vi "ActorPlugin-001-CreateInstructions.vi"(0 "FTW Actor Instance Configuration":string="{\n  \"Identity\": \"ActorName\",\n  \"InboxAddress\": \"tcp://127.0.0.1:*\",\n  \"PublisherAddress\": \"tcp://127.0.0.1:*\",\n  \"DebugEnableInboxLogging\": false,\n  \"DebugEnableJobLogging\": false,\n  \"DebugShowPanel\": false\n}", 11 "Error in":errorcluster) -> (15 "Error":errorcluster)   [LabVIEW 2013, in "ERP-CreateInstructions.lvclass"]
uses:
  Actors/ERP-Create Instructions Plugin/ERP-CreateInstructions/ERP-CreateInstructions.lvclass
  Actors/ERP-Create Instructions Plugin/Instruction Controls/Cntrl-CreateManuInstruction.ctl
  Actors/ERP-Create Instructions Plugin/Instruction Controls/Cntrl-UpdateInstruction.ctl
  Actors/ERP-Create Instructions Plugin/Instruction Controls/Cntrl-CreateInspectInstruction.ctl
  Actors/ERP-Create Instructions Plugin/Instruction Controls/Cntrl-CreateGeneralInstruction.ctl
  Actors/ERP-Create Instructions Plugin/Instruction Controls/Cntrl-Manufacturing.ctl
  Actors/ERP-Create Instructions Plugin/Instruction Controls/Cntrl-Inspection.ctl
  Actors/ERP-Create Instructions Plugin/Instruction Controls/Cntrl-GenericCenter.ctl
  Actors/ERP-Create Instructions Plugin/Instruction Controls/Cntrl-ClearStep.ctl
  Actors/ERP-Create Instructions Plugin/Instruction Controls/Cntrl-LoadInstruction.ctl
  Actors/ERP-Create Instructions Plugin/Instruction Controls/Cntrl-ChooseGeneralStep.ctl
  Actors/ERP-Create Instructions Plugin/Instruction Controls/Cntrl-RefreshTree.ctl
  Actors/ERP-Create Instructions Plugin/Instruction Controls/Cntrl-ClearAllSteps.ctl
  Actors/ERP-Create Instructions Plugin/Instruction Controls/Cntrl-DeleteTreeItem.ctl
  Actors/ERP-Create Instructions Plugin/ERP-CreateInstructions/ERP-CreateInstructions.lvclass/ERP-CreateInstructions.ctl
  ftw-dataflow/Actor/src/Instance/FTW-ActorInstance.lvclass
  ftw-dataflow/Actor/src/Message/Request/FTW-Message-IncomingRequest.lvclass
  ERP-ConfigPageNewFeather/PCert-ConfigPageNF.lvclass
  <vilib>/addons/_LabVIEW Style Book/Utilities/Style Book Utilities.lvlib
panel:
  in  "Manufacturing Center":T1
  in  "Inspection Center":T2
  in  "Generic Instruction Center":T3
  in  "Stop Button":bool
  in  "Tab Control -Main":T4(tab)
  in  "Refresh Manufacturing Tree":T5
  in  "Clear Manu Step#":T6
  in  "Go Back A Step - Manu":bool
  in  "Go to next step-Manu":bool
  in  "Manufacturing Tab Instructions":T7(tab)
  in  "Manufacturing-Part Number":string
  in  "Manufacturing-Mat":T8={"Get Material Instruction"="", "Path for Picture Material"=path "", "Path for Picture Material 2"=path "", "Path for Picture Material 3"=path "", "Path for Picture Material 4"=path "", "Path for Picture Material 5"=path "", "Path for Picture Material 6"=path "", "Path for Picture Material 7"=path "", "Step Number"="1", "General Instruction"=""}
  in  "Manufacturing-VisualInsp":T9={"Visual Inspection Instruction"="", "Path for Picture VisualInsp"=path "", "Path for Picture VisualInsp 2"=path "", "Path for Picture VisualInsp 3"=path "", "Path for Picture VisualInsp 4"=path "", "Path for Picture VisualInsp 5"=path "", "Path for Picture VisualInsp 6"=path "", "Path for Picture VisualInsp 7"=path "", "Step Number"="2", "General Instruction"=""}
  in  "Manufacturing-Assemble":T10={"Assemble Material as Required"="", "Path for Picture Assemble"=path "", "Path for Picture Assemble 2"=path "", "Path for Picture Assemble 3"=path "", "Path for Picture Assemble 4"=path "", "Path for Picture Assemble 5"=path "", "Path for Picture Assemble 6"=path "", "Path for Picture Assemble 7"=path "", "Step Number"="3", "General Instruction"=""}
  in  "Manufacturing-Laser":T11={"Laser Cutting Instructions"="", "Path for Picture Laser Cutting"=path "", "Path for Picture Laser Cutting 2"=path "", "Path for Picture Laser Cutting 3"=path "", "Path for Picture Laser Cutting 4"=path "", "Path for Picture Laser Cutting 5"=path "", "Path for Picture Laser Cutting 6"=path "", "Path for Picture Laser Cutting 7"=path "", "Step Number"="4", "General Instruction"=""}
  in  "Manufacturing-Cleaning":T12={"Cleaning Instructions"="", "Path for Picture Cleaning"=path "", "Path for Picture Cleaning 2"=path "", "Path for Picture Cleaning 3"=path "", "Path for Picture Cleaning 4"=path "", "Path for Picture Cleaning 5"=path "", "Path for Picture Cleaning 6"=path "", "Path for Picture Cleaning 7"=path "", "Step Number"="5", "General Instruction"=""}
  in  "Manufacturing-Label":T13={"Label Instructions"="", "Path for Picture Label"=path "", "Path for Picture Label 2"=path "", "Path for Picture Label 3"=path "", "Path for Picture Label 4"=path "", "Path for Picture Label 5"=path "", "Path for Picture Label 6"=path "", "Path for Picture Label 7"=path "", "Step Number"="6", "General Instruction"=""}
  in  "Manufacturing Tree - Instruction Sets":string(tree)
  in  "Create Manufacturing Instruction":T14
  in  "Update Manufacturing Instruction":T15
  in  "Load Manufacturing Instruction":T16
  in  "Choose General Step\nManufacturing":T17
  in  "Clear All Manu\nSteps":T18
  in  "Delete Manufacturing Instruction":T19
  in  "Delete Inspection Instruction":T19
  in  "Clear All Inspection\nSteps":T18
  in  "Refresh Inspection Tree":T5
  in  "Inspection Tab Instructions":T20(tab)
  in  "Inspection Part Number":string caption="Part Number Inspection"
  in  "Inspect-Visually Inspect":T21={"Visual Inspection Instruction"="", "Path for Picture Material"=path "", "Path for Picture Material 2"=path "", "Path for Picture Material 3"=path "", "Path for Picture Material 4"=path "", "Path for Picture Material 5"=path "", "Path for Picture Material 6"=path "", "Path for Picture Material 7"=path "", "Step Number"="1", "General Instruction"=""}
  in  "Inspect-Certified Material":T22={"Certified Material Instruction"="", "Path for Picture VisualInsp"=path "", "Path for Picture VisualInsp 2"=path "", "Path for Picture VisualInsp 3"=path "", "Path for Picture VisualInsp 4"=path "", "Path for Picture VisualInsp 5"=path "", "Path for Picture VisualInsp 6"=path "", "Path for Picture VisualInsp 7"=path "", "Step Number"="2", "General Instruction"=""}
  in  "Inspect-XY Dimensions":T23={"XY Dimensions Instructions"="", "Path for Picture Assemble"=path "", "Path for Picture Assemble 2"=path "", "Path for Picture Assemble 3"=path "", "Path for Picture Assemble 4"=path "", "Path for Picture Assemble 5"=path "", "Path for Picture Assemble 6"=path "", "Path for Picture Assemble 7"=path "", "Step Number"="3", "General Instruction"=""}
  in  "Inspect-Measure Create Cert":T24={"Measure and Create Certification Instructions"="", "Path for Picture Laser Cutting"=path "", "Path for Picture Laser Cutting 2"=path "", "Path for Picture Laser Cutting 3"=path "", "Path for Picture Laser Cutting 4"=path "", "Path for Picture Laser Cutting 5"=path "", "Path for Picture Laser Cutting 6"=path "", "Path for Picture Laser Cutting 7"=path "", "Step Number"="4", "General Instruction"=""}
  in  "Inspect-Qty P/F":T25={"Quantity Passed or Failed Instructions"="", "Path for Picture Cleaning"=path "", "Path for Picture Cleaning 2"=path "", "Path for Picture Cleaning 3"=path "", "Path for Picture Cleaning 4"=path "", "Path for Picture Cleaning 5"=path "", "Path for Picture Cleaning 6"=path "", "Path for Picture Cleaning 7"=path "", "Step Number"="5", "General Instruction"=""}
  in  "Inspect-Inspect Labels":T26={"Inspect Label Instructions"="", "Path for Picture Label"=path "", "Path for Picture Label 2"=path "", "Path for Picture Label 3"=path "", "Path for Picture Label 4"=path "", "Path for Picture Label 5"=path "", "Path for Picture Label 6"=path "", "Path for Picture Label 7"=path "", "Step Number"="6", "General Instruction"=""}
  in  "Inspection Tree - Instruction Sets":string(tree)
  in  "Go to next step-Insp":bool
  in  "Go Back A Step - Insp":bool
  in  "Create Inspection Instruction":T27
  in  "Clear Inspect Step#":T6
  in  "Load Inspection Instruction":T16
  in  "Update Inspection Instruction":T15
  in  "Choose General Step\nInspection":T17
  in  "Step Number*":dbl
  in  "General Process Name*":string
  in  "General Tree - Instruction Sets":string(tree)
  in  "Create General Instruction":T28
  in  "General Step Instruction":T29
  in  "Clear General Step#":T6
  in  "Refresh General Tree":T5
  in  "Update General Instruction":T15
  in  "Delete General Instruction":T19
  # "Instruction Controls"
  # "Inputs"
  # "Outputs"
  # "Please Enter the Part Number"
  # "Enter Instruction for Get Material"
  # "Enter Instruction Visual Inspection"
  # "Enter Instruction for Assemble Material as Required"
  # "Enter Instruction for Laser Cutting"
  # "Enter Instruction for Cleaning"
  # "Enter Instruction for Label"
  # "Please Enter the Part Number"
  # "Enter Instruction for Visually Inspect"
  # "Enter Instruction Verify Certified Material Was Used"
  # "Enter Instruction for Verify XY Dimensions"
  # "Enter Instruction Measure: Create Certification if Required"
  # "Enter Instruction For Verify Quantity Passed or Failed"
  # "Enter Instruction for Label Inspection"
  # "General Instuctions"
  # "*=Required"
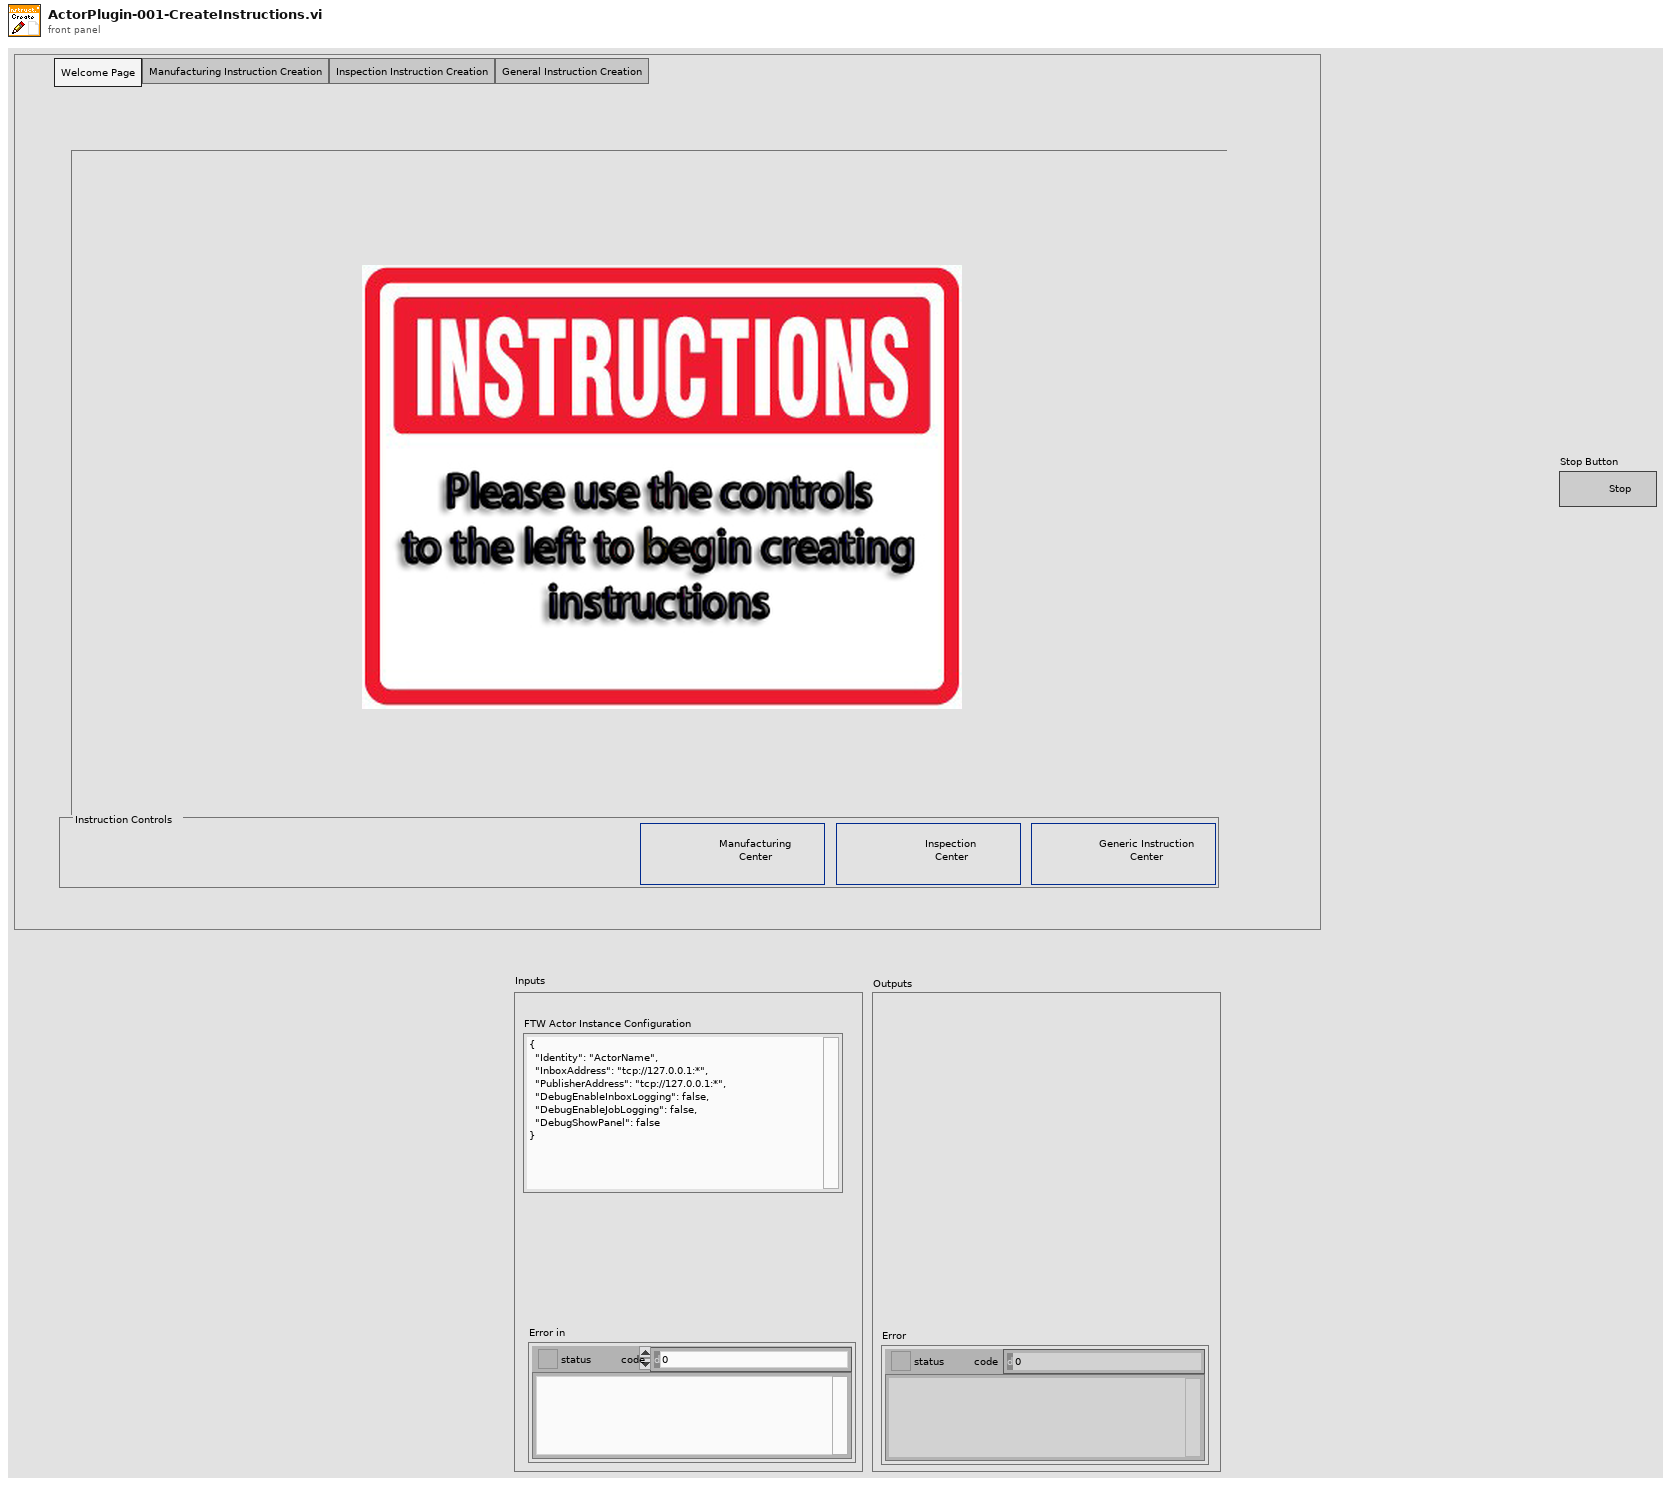
[diagram p1: front panel]
types:
  T1 = typedef "Cntrl-Manufacturing.ctl" = bool
  T2 = typedef "Cntrl-Inspection.ctl" = bool
  T3 = typedef "Cntrl-GenericCenter.ctl" = bool
  T4 = enum32{"Welcome Page", "Manufacturing Instruction Creation", "Inspection Instruction Creation", "General Instruction Creation"}
  T5 = typedef "Cntrl-RefreshTree.ctl" = bool
  T6 = typedef "Cntrl-ClearStep.ctl" = bool
  T7 = enum32{"Enter Part Number", "Get Material Instructions", "Visual Inspection Instruction", "Assemble Material as Required", "Laser Cutting Instructions", "Cleaning Instructions", "Label Instructions"}
  T8 = cluster{"Get Material Instruction":string, "Path for Picture Material":path, "Path for Picture Material 2":path, "Path for Picture Material 3":path, "Path for Picture Material 4":path, "Path for Picture Material 5":path, "Path for Picture Material 6":path, "Path for Picture Material 7":path, "Step Number":string, "General Instruction":string}
  T9 = cluster{"Visual Inspection Instruction":string, "Path for Picture VisualInsp":path, "Path for Picture VisualInsp 2":path, "Path for Picture VisualInsp 3":path, "Path for Picture VisualInsp 4":path, "Path for Picture VisualInsp 5":path, "Path for Picture VisualInsp 6":path, "Path for Picture VisualInsp 7":path, "Step Number":string, "General Instruction":string}
  T10 = cluster{"Assemble Material as Required":string, "Path for Picture Assemble":path, "Path for Picture Assemble 2":path, "Path for Picture Assemble 3":path, "Path for Picture Assemble 4":path, "Path for Picture Assemble 5":path, "Path for Picture Assemble 6":path, "Path for Picture Assemble 7":path, "Step Number":string, "General Instruction":string}
  T11 = cluster{"Laser Cutting Instructions":string, "Path for Picture Laser Cutting":path, "Path for Picture Laser Cutting 2":path, "Path for Picture Laser Cutting 3":path, "Path for Picture Laser Cutting 4":path, "Path for Picture Laser Cutting 5":path, "Path for Picture Laser Cutting 6":path, "Path for Picture Laser Cutting 7":path, "Step Number":string, "General Instruction":string}
  T12 = cluster{"Cleaning Instructions":string, "Path for Picture Cleaning":path, "Path for Picture Cleaning 2":path, "Path for Picture Cleaning 3":path, "Path for Picture Cleaning 4":path, "Path for Picture Cleaning 5":path, "Path for Picture Cleaning 6":path, "Path for Picture Cleaning 7":path, "Step Number":string, "General Instruction":string}
  T13 = cluster{"Label Instructions":string, "Path for Picture Label":path, "Path for Picture Label 2":path, "Path for Picture Label 3":path, "Path for Picture Label 4":path, "Path for Picture Label 5":path, "Path for Picture Label 6":path, "Path for Picture Label 7":path, "Step Number":string, "General Instruction":string}
  T14 = typedef "Cntrl-CreateManuInstruction.ctl" = bool
  T15 = typedef "Cntrl-UpdateInstruction.ctl" = bool
  T16 = typedef "Cntrl-LoadInstruction.ctl" = bool
  T17 = typedef "Cntrl-ChooseGeneralStep.ctl" = bool
  T18 = typedef "Cntrl-ClearAllSteps.ctl" = bool
  T19 = typedef "Cntrl-DeleteTreeItem.ctl" = bool
  T20 = enum32{"Enter Part Number", "Visually Inspect", "Certified Material", "XY Dimensions", "Measure Create Cert", "Quantity Passed or Failed", "Inspect Labels"}
  T21 = cluster{"Visual Inspection Instruction":string, "Path for Picture Material":path, "Path for Picture Material 2":path, "Path for Picture Material 3":path, "Path for Picture Material 4":path, "Path for Picture Material 5":path, "Path for Picture Material 6":path, "Path for Picture Material 7":path, "Step Number":string, "General Instruction":string}
  T22 = cluster{"Certified Material Instruction":string, "Path for Picture VisualInsp":path, "Path for Picture VisualInsp 2":path, "Path for Picture VisualInsp 3":path, "Path for Picture VisualInsp 4":path, "Path for Picture VisualInsp 5":path, "Path for Picture VisualInsp 6":path, "Path for Picture VisualInsp 7":path, "Step Number":string, "General Instruction":string}
  T23 = cluster{"XY Dimensions Instructions":string, "Path for Picture Assemble":path, "Path for Picture Assemble 2":path, "Path for Picture Assemble 3":path, "Path for Picture Assemble 4":path, "Path for Picture Assemble 5":path, "Path for Picture Assemble 6":path, "Path for Picture Assemble 7":path, "Step Number":string, "General Instruction":string}
  T24 = cluster{"Measure and Create Certification Instructions":string, "Path for Picture Laser Cutting":path, "Path for Picture Laser Cutting 2":path, "Path for Picture Laser Cutting 3":path, "Path for Picture Laser Cutting 4":path, "Path for Picture Laser Cutting 5":path, "Path for Picture Laser Cutting 6":path, "Path for Picture Laser Cutting 7":path, "Step Number":string, "General Instruction":string}
  T25 = cluster{"Quantity Passed or Failed Instructions":string, "Path for Picture Cleaning":path, "Path for Picture Cleaning 2":path, "Path for Picture Cleaning 3":path, "Path for Picture Cleaning 4":path, "Path for Picture Cleaning 5":path, "Path for Picture Cleaning 6":path, "Path for Picture Cleaning 7":path, "Step Number":string, "General Instruction":string}
  T26 = cluster{"Inspect Label Instructions":string, "Path for Picture Label":path, "Path for Picture Label 2":path, "Path for Picture Label 3":path, "Path for Picture Label 4":path, "Path for Picture Label 5":path, "Path for Picture Label 6":path, "Path for Picture Label 7":path, "Step Number":string, "General Instruction":string}
  T27 = typedef "Cntrl-CreateInspectInstruction.ctl" = bool
  T28 = typedef "Cntrl-CreateGeneralInstruction.ctl" = bool
  T29 = cluster{"General Instruction Step":string, "Path for Picture General":path, "Path for Picture General 2":path, "Path for Picture General 3":path, "Path for Picture General 4":path, "Path for Picture General 5":path, "Path for Picture General 6":path, "Path for Picture General 7":path}
  T30 = cluster{"Manufacturing-Part Number":string, dbl, "Manufacturing-Label":cluster{"Label Instructions":string, "Path for Picture Label":path, "Path for Picture Label 2":path, "Path for Picture Label 3":path, "Path for Picture Label 4":path, "Path for Picture Label 5":path, "Path for Picture Label 6":path, "Path for Picture Label 7":path}}
  T31 = enum32{"Welcome Page", "Manufacturing Instruction Creation", "Inspection Instruction Creation"}
  T32 = cluster{"Manufacturing-Part Number":string, "Array of Cluster Data":cluster{"Label Instructions":string, "Path for Picture Label":path, "Path for Picture Label 2":path, "Path for Picture Label 3":path, "Path for Picture Label 4":path, "Path for Picture Label 5":path, "Path for Picture Label 6":path, "Path for Picture Label 7":path, "Label Instructions 2":string, "Label Instructions 3":string}[], "Type of Insert":i32}
  T33 = cluster{"Manufacturing-Part Number":string, "Step Number":dbl, "Gernal Cluster Data":cluster{"Label Instructions":string, "Path for Picture Label":path, "Path for Picture Label 2":path, "Path for Picture Label 3":path, "Path for Picture Label 4":path, "Path for Picture Label 5":path, "Path for Picture Label 6":path, "Path for Picture Label 7":path}, "Type of Insert":i32}
  T34 = cluster{"Label Instructions":string, "Path for Picture Label":path, "Path for Picture Label 2":path, "Path for Picture Label 3":path, "Path for Picture Label 4":path, "Path for Picture Label 5":path, "Path for Picture Label 6":path, "Path for Picture Label 7":path, "Step Number":string, "General Instruction":string}[]
  T35 = cluster{"Value":string, cluster{"Label Instructions":string, "Path for Picture Label":path, "Path for Picture Label 2":path, "Path for Picture Label 3":path, "Path for Picture Label 4":path, "Path for Picture Label 5":path, "Path for Picture Label 6":path, "Path for Picture Label 7":path, "Step Number":string, "General Instruction":string}[]}
  T36 = cluster{"Inspect Label Instructions":string, "Path for Picture Label":path, "Path for Picture Label 2":path, "Path for Picture Label 3":path, "Path for Picture Label 4":path, "Path for Picture Label 5":path, "Path for Picture Label 6":path, "Path for Picture Label 7":path, "Step Number":string, "General Instruction":string}[]
  T37 = cluster{"Value":string, cluster{"Inspect Label Instructions":string, "Path for Picture Label":path, "Path for Picture Label 2":path, "Path for Picture Label 3":path, "Path for Picture Label 4":path, "Path for Picture Label 5":path, "Path for Picture Label 6":path, "Path for Picture Label 7":path, "Step Number":string, "General Instruction":string}[]}
  T38 = cluster{"Incoming Requests":refnum<event-registration>, "Additional Registration Types":refnum<event-registration>}
  T39 = cluster{"Label Instructions":string, "Path for Picture Label":path, "Path for Picture Label 2":path, "Path for Picture Label 3":path, "Path for Picture Label 4":path, "Path for Picture Label 5":path, "Path for Picture Label 6":path, "Path for Picture Label 7":path, "Step Number":string, "Generall Instruction":string}[]
  T40 = cluster{"Label Instructions":string, "Path for Picture Label":path, "Path for Picture Label 2":path, "Path for Picture Label 3":path, "Path for Picture Label 4":path, "Path for Picture Label 5":path, "Path for Picture Label 6":path, "Path for Picture Label 7":path}
  T41 = cluster{"Instructions":string, "Picture Path 1":path, "Picture Path 2":path, "Picture Path 3":path, "Picture Path 4":path, "Picture Path 5":path, "Picture Path 6":path, "Picture Path 7":path, "Step":string, "General Instruction":string}[]
  T42 = cluster{"Instructions":string, "Picture Path 1":path, "Picture Path 2":path, "Picture Path 3":path, "Picture Path 4":path, "Picture Path 5":path, "Picture Path 6":path, "Picture Path 7":path, "Step":string, "General Instrucion":string}
  T43 = cluster{"Instructions":string, "Picture Path 1":path, "Picture Path 2":path, "Picture Path 3":path, "Picture Path 4":path, "Picture Path 5":path, "Picture Path 6":path, "Picture Path 7":path, "Step Instruction":string, "General Instruction":string}
  T44 = cluster{"Instructions":string, "Picture Path 1":path, "Picture Path 2":path, "Picture Path 3":path, "Picture Path 4":path, "Picture Path 5":path, "Picture Path 6":path, "Picture Path 7":path}
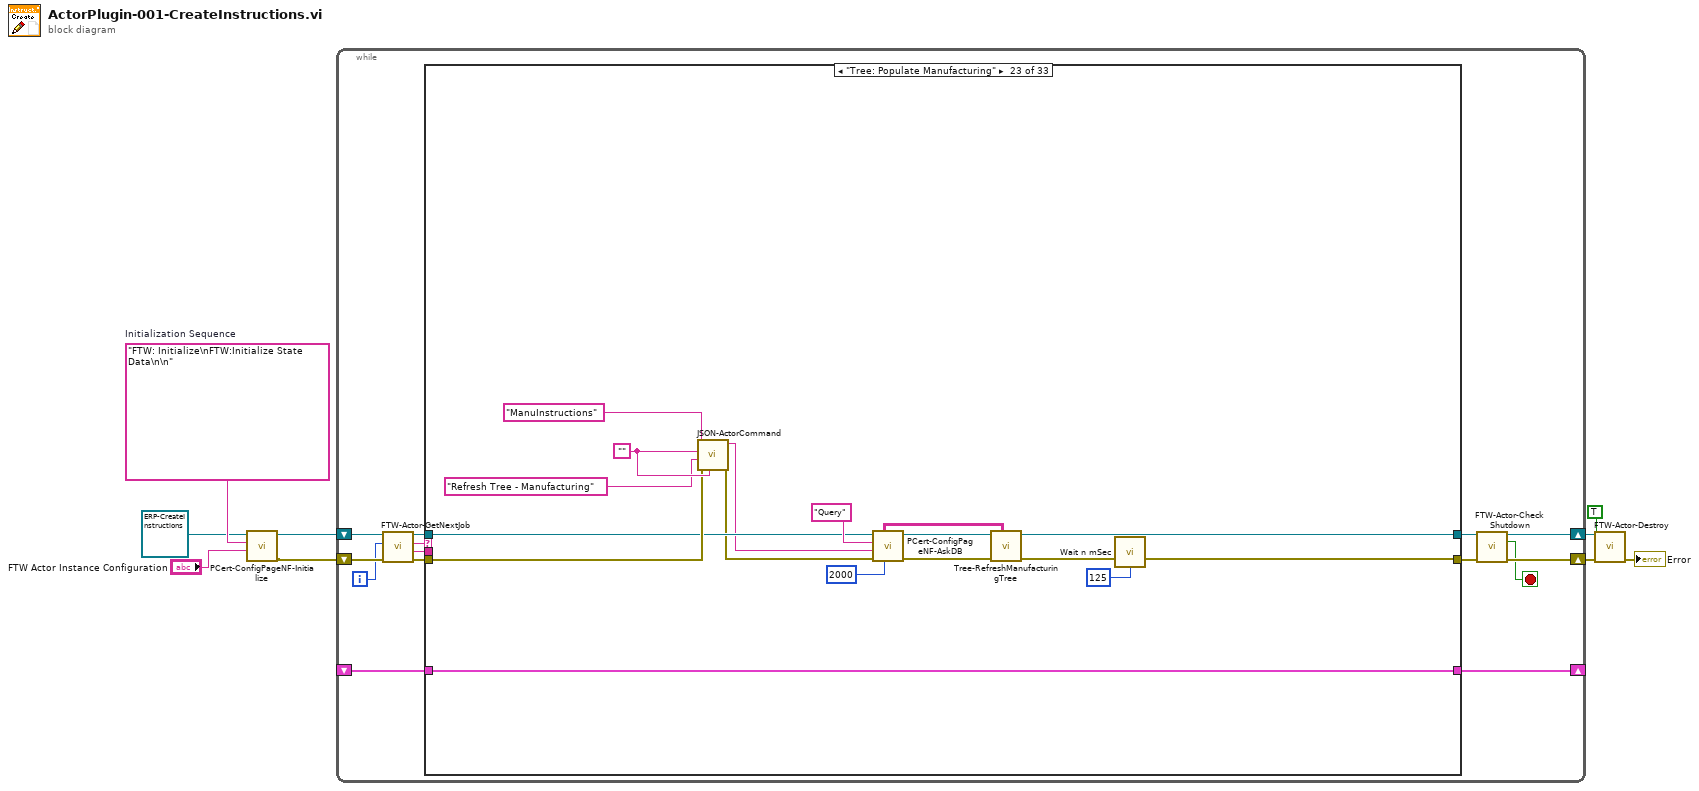
[diagram p0: block diagram]
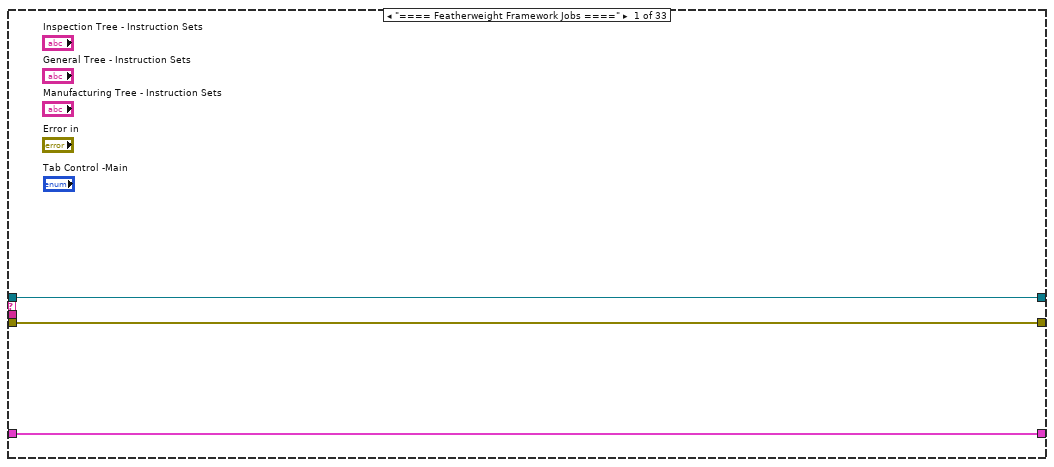
[diagram p2: hidden frame]
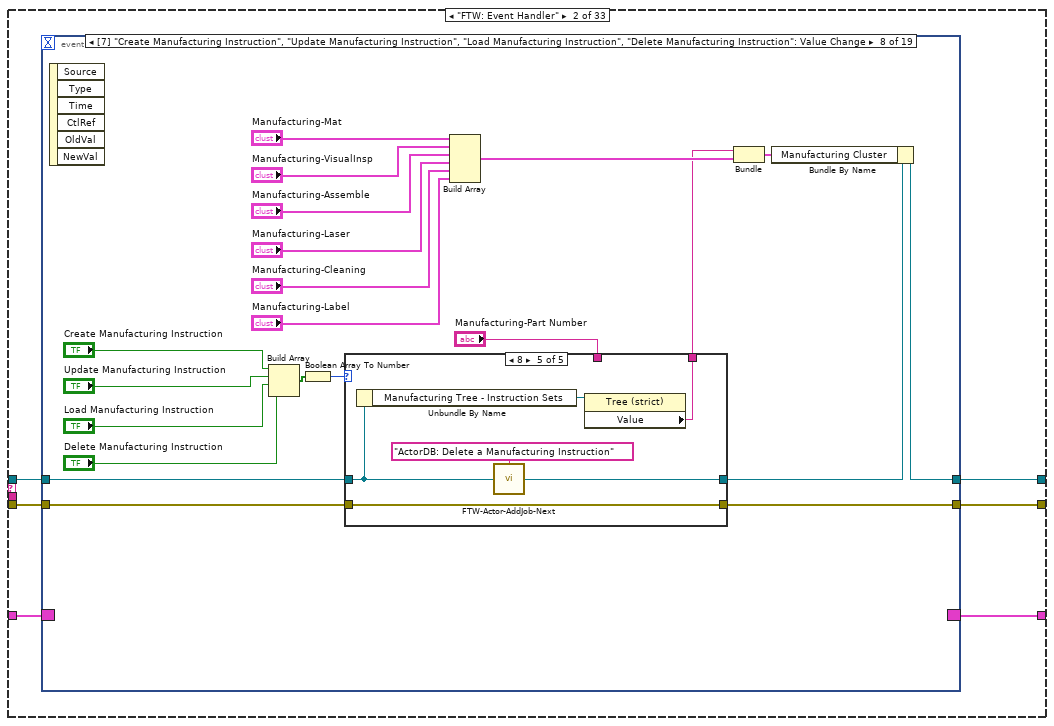
[diagram p3: hidden frame]
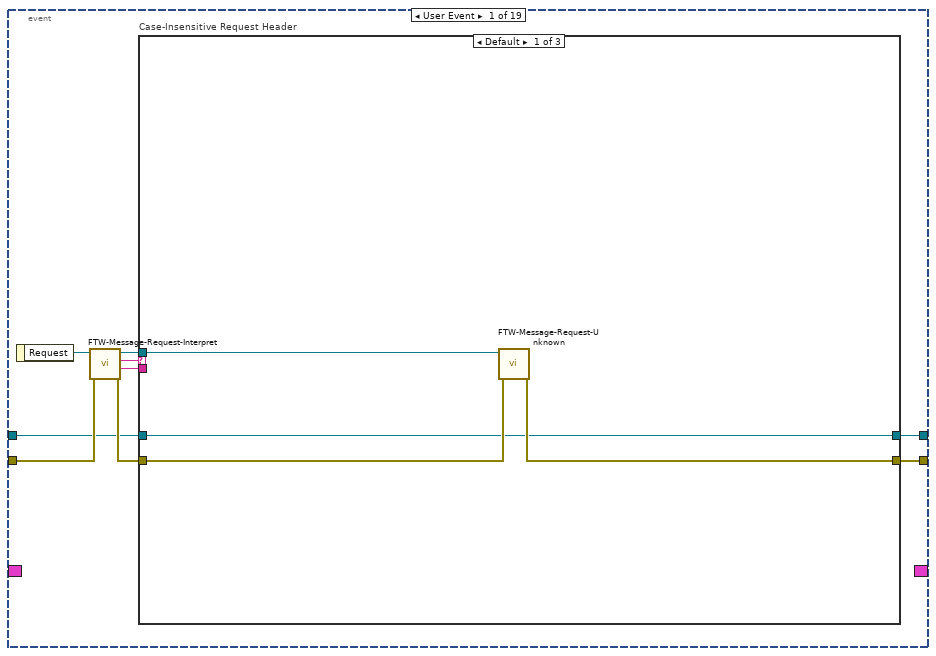
[diagram p4: hidden frame]
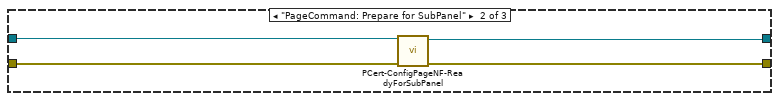
[diagram p5: hidden frame]
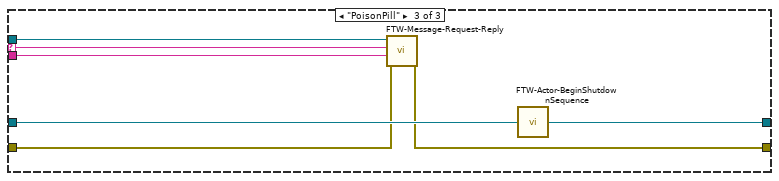
[diagram p6: hidden frame]
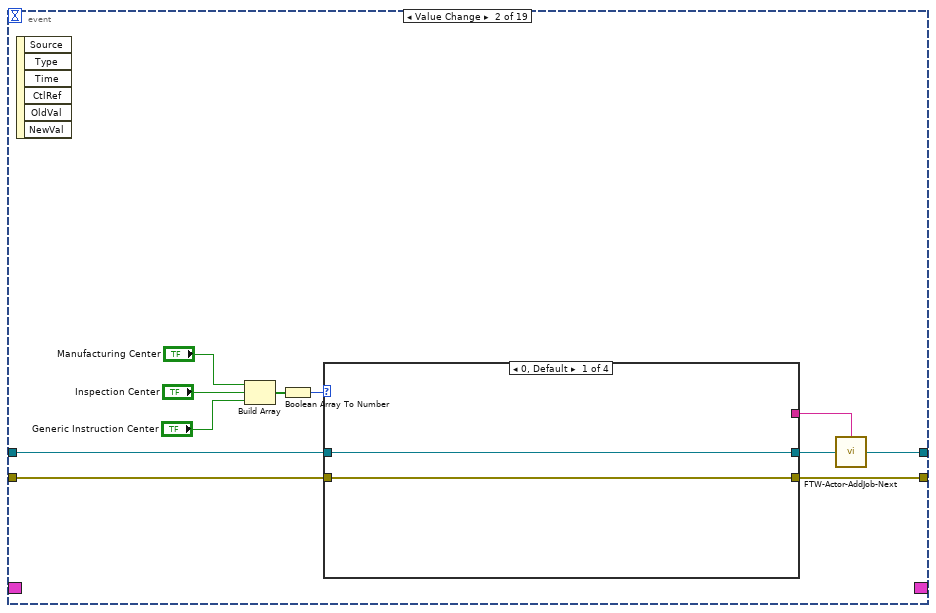
[diagram p7: hidden frame]
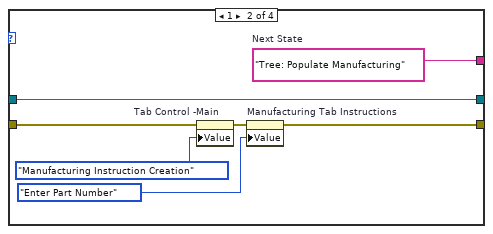
[diagram p8: hidden frame]
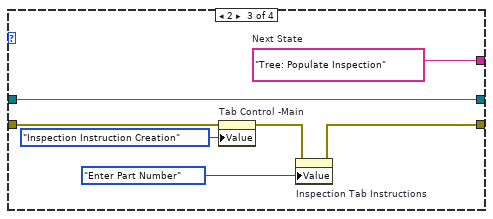
[diagram p9: hidden frame]
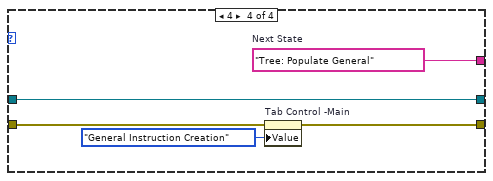
[diagram p10: hidden frame]
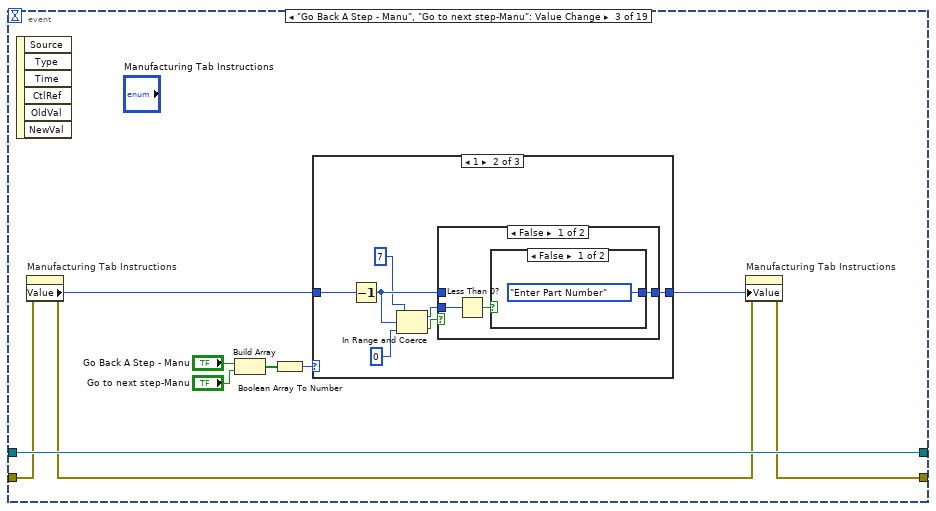
[diagram p11: hidden frame]
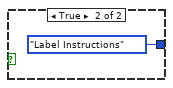
[diagram p13: hidden frame]
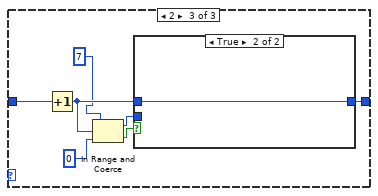
[diagram p15: hidden frame]
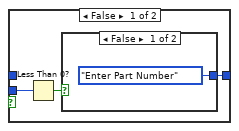
[diagram p16: hidden frame]
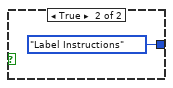
[diagram p17: hidden frame]
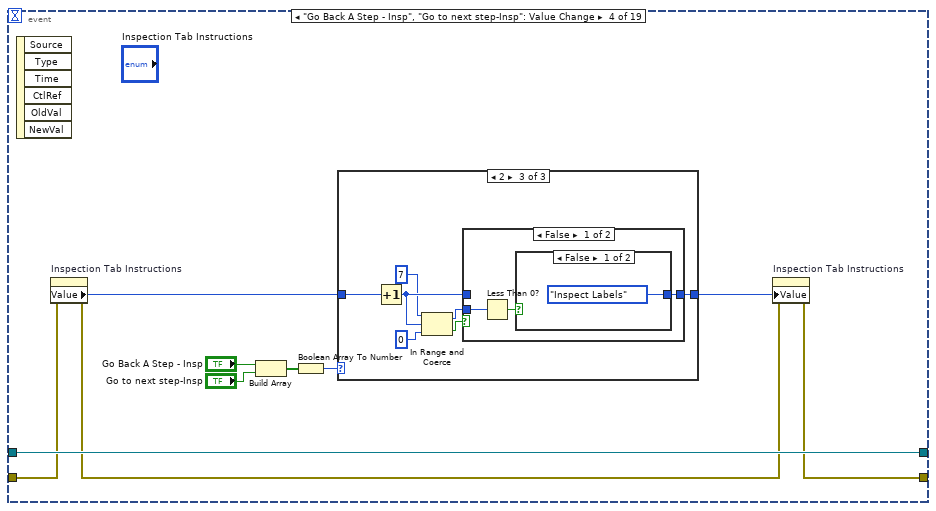
[diagram p18: hidden frame]
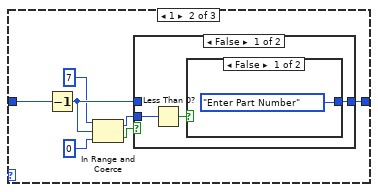
[diagram p20: hidden frame]
diagram:
  w6 = "FTW: Initialize\nFTW:Initialize State Data\n\n"  # Initialization Sequence
  n1 = call-dynamic "PCert-ConfigPageNF-Initialize.vi"("FTW Actor Instance Configuration"="FTW Actor Instance Configuration", "Initialization Job Sequence"=w6, "ERP-ConfigPageNF.lvclass"=refnum<class "ERP-CreateInstructions.lvclass"> refnum ("ERP-CreateInstructions.lvclass")) -> ("error out"=w4:errorcluster, "ERP-ConfigPageNF out"=w5:refnum<class "ERP-CreateInstructions.lvclass">)  [unwired: 7 in]
  n2 = while {
    shift-right: [w13] -> w8
    shift-left: w4 -> [w20]
    shift-right: [w10] -> _
    shift-left: _ -> [w23]
    shift-right: [w15] -> w9
    shift-left: w5 -> [w22]
    i -> [w11]
    stop <- w12 stop-if-true
    n3 = call "FTW-Actor-GetNextJob.vi"("error in"=w20, "Jobs Performed"=w11, "FTW Actor Instance"=w22) -> ("error out"=w19:errorcluster, "Job Data"=w17:string, "Job Name"=w18:string, "FTW Actor Instance out"=w21:refnum<class "ERP-CreateInstructions.lvclass">)  [unwired: 5 in]
    n4 = case shown="\"Tree: Populate Manufacturing\"" w18 {
      selector: w18 -> [_ _ _ _ _ w435 _ _ _ _ _ _ _ _ _ _ _ _ _ _ _ _ _ _ _ _ _ _ _ _ _ _ _]
      tunnel: [w25 w32 w418 w428 w430 w438 w446 w452 w457 w461 w465 w491 w510 w534 w558 w580 w606 w639 w682 w698 w723 w755 w757 w774 w791 w808 w811 w814 w873 w919 w931 w945 w997] -> w14
      tunnel: w19 -> [w25 w31 w410 w428 w432 w439 w443 w452 w457 w461 w462 w485 w519 w532 w556 w590 w615 w648 w684 w712 w733 w755 w769 w786 w803 w808 w811 w821 w871 w926 w931 w936 w1001]
      tunnel: w23 -> [w26 w27 _ w429 w434 w440 w448 w453 w458 w460 w484 w507 w531 w555 w579 w604 w616 w650 w697 w722 w751 w756 w773 w790 w807 w810 w813 w822 w874 w929 w932 w948 w1009]
      tunnel: [w26 w30 w412 w429 w434 w440 w448 w453 w458 w460 w484 w507 w531 w555 w579 w604 w616 w650 w697 w722 w751 w756 w773 w790 w807 w810 w813 w822 w874 w929 w932 w948 w1009] -> w10
      tunnel: w17 -> [_ _ _ _ _ _ _ _ _ _ _ _ _ _ _ _ _ _ _ _ _ _ _ _ _ _ _ _ _ _ _ _ _]
      tunnel: [w24 w29 w419 w425 w431 w436 w441 w450 w455 w459 w466 w492 w511 w535 w559 w581 w613 w646 w683 w699 w727 w754 w760 w777 w794 w809 w812 w818 w868 w928 w930 w944 w998] -> w16
      tunnel: w21 -> [w24 w28 w417 w427 w433 w437 w444 w451 w456 w459 w463 w486 w515 w533 w557 w587 w614 w647 w681 w711 w746 w754 w766 w783 w800 w809 w812 w820 w872 w927 w930 w937 w1002]
      frame "==== Featherweight Framework Jobs ====" {
      }
      frame "FTW: Event Handler" {
        n5 = event shown="[7] \"Create Manufacturing Instruction\", \"Update Manufacturing Instruction\", \"Load Manufacturing Instruction\", \"Delete Manufacturing Instruction\": Value Change" {
          selector: w27 -> [_ _ _ _ _ _ _ _ _ _ _ _ _ _ _ _ _ _ _]
          dyn-events: [_ _ _ _ _ _ _ _ _ _ _ _ _ _ _ _ _ _ _] -> w30
          timeout: _ -> [_ _ _ _ _ _ _ _ _ _ _ _ _ _ _ _ _ _ _]
          tunnel: [w38 w66 w97 w132 w163 w182 w201 w219 w254 w258 w273 w304 w311 w312 w336 w366 w400 w403 w406] -> w32
          tunnel: w31 -> [w39 w67 w96 w134 w166 w185 w202 w226 w254 w258 w274 w304 w311 w313 w337 w371 w400 w403 w406]
          tunnel: [w37 w58 w98 w135 w167 w186 w205 w210 w251 w255 w271 w305 w308 w314 w335 w373 w397 w401 w404] -> w29
          tunnel: w28 -> [w36 w62 w98 w135 w167 w186 w205 w225 w252 w256 w275 w306 w309 w315 w335 w372 w398 w402 w405]
          event User Event {
            n6 = event-data() -> ("Request"=w40:refnum<class "FTW-Message-IncomingRequest.lvclass">)  [unwired: 1 in]
            n7 = call "FTW-Message-Request-Interpret.vi"("error in"=w39, "FTW Incoming Request"=w40) -> ("error out"=w41:errorcluster, "Request Body"=w34:string, "Request Header"=w35:string, "FTW Incoming Request out"=w33:refnum<class "FTW-Message-IncomingRequest.lvclass">)  [unwired: 6 in]
            n8 = case "Case-Insensitive Request Header" shown="Default" w35 {
              selector: w35 -> [_ _ w52]
              tunnel: [w44 w46 w50] -> w38
              tunnel: w41 -> [w45 w47 w51]
              tunnel: [w42 w48 w56] -> w37
              tunnel: w36 -> [w42 w49 w55]
              tunnel: w34 -> [_ _ w53]
              tunnel: w33 -> [w43 _ w54]
              frame Default {
                n9 = call "FTW-Message-Request-Unknown.vi"("error in"=w45, "FTW Incoming Request"=w43) -> ("error out"=w44:errorcluster)  [unwired: 9 in]
              }
              frame "PageCommand: Prepare for SubPanel" {
                n10 = call "PCert-ConfigPageNF-ReadyForSubPanel.vi"("error in (no error)"=w47, "ERP-ConfigPageNF in"=w49) -> ("error out"=w46:errorcluster, "ERP-ConfigPageNF out"=w48:refnum<class "ERP-CreateInstructions.lvclass">)  [unwired: 8 in]
              }
              frame "PoisonPill" {
                n11 = call "FTW-Message-Request-Reply.vi"("error in"=w51, "Response Body"=w53, "Response Header"=w52, "FTW Incoming Request"=w54) -> ("error out"=w50:errorcluster)  [unwired: 6 in, 1 out]
                n12 = call "FTW-Actor-BeginShutdownSequence.vi"("FTW Actor Instance"=w55) -> ("FTW Actor Instance out"=w56:refnum<class "ERP-CreateInstructions.lvclass">)  [unwired: 3 in]
              }
            }
          }
          event Value Change {
            n13 = event-data() -> ()  [unwired: 1 in, 6 out]
            n14 = Build Array("Manufacturing Center", "Inspection Center", "Generic Instruction Center") -> (w61:T3[])
            n15 = Boolean Array To Number(Boolean array=w61) -> (number=w60:u32)
            n16 = case shown="0, Default" w60 {
              tunnel: w67 -> [w68 w76 w83 w88]
              tunnel: [w68 w71 w77 w87] -> w66
              tunnel: w62 -> [w69 w74 w81 w85]
              tunnel: [w69 w74 w81 w85] -> w59
              tunnel: [_ w70 w80 w84] -> w57
              frame 0, Default {
              }
              frame 1 {
                w70 = "Tree: Populate Manufacturing"  # Next State
                n17 = property on="Tab Control -Main" class="TabCtl (strict)"(error in=w76, "Value"=T4."Manufacturing Instruction Creation" ("Tab Control -Main")) -> (error out=w72:errorcluster)  [unwired: 1 in, 1 out]
                n18 = property on="Manufacturing Tab Instructions" class="TabCtl (strict)"(error in=w72, "Value"=T7."Enter Part Number" ("Manufacturing Tab Instructions")) -> (error out=w71:errorcluster)  [unwired: 1 in, 1 out]
              }
              frame 2 {
                w80 = "Tree: Populate Inspection"  # Next State
                n19 = property on="Tab Control -Main" class="TabCtl (strict)"(error in=w83, "Value"=T4."Inspection Instruction Creation" ("Tab Control -Main")) -> (error out=w78:errorcluster)  [unwired: 1 in, 1 out]
                n20 = property on="Inspection Tab Instructions" class="TabCtl (strict)"(error in=w78, "Value"=T20."Enter Part Number" ("Inspection Tab Instructions")) -> (error out=w77:errorcluster)  [unwired: 1 in, 1 out]
              }
              frame 4 {
                w84 = "Tree: Populate General"  # Next State
                n21 = property on="Tab Control -Main" class="TabCtl (strict)"(error in=w88, "Value"=T4."General Instruction Creation" ("Tab Control -Main")) -> (error out=w87:errorcluster)  [unwired: 1 in, 1 out]
              }
            }
            n22 = call "FTW-Actor-AddJob-Next.vi"("Add Next in Job Queue"=w57, "FTW Actor Instance"=w59) -> ("FTW Actor Instance out"=w58:refnum<class "ERP-CreateInstructions.lvclass">)  [unwired: 2 in]
          }
          event "Go Back A Step - Manu", "Go to next step-Manu": Value Change {
            n23 = event-data() -> ()  [unwired: 1 in, 6 out]
            n24 = property on="Manufacturing Tab Instructions" class="TabCtl (strict)"(error in=w96) -> (error out=w95:errorcluster, "Value"=w90:T7)  [unwired: 1 in, 1 out]
            n25 = Build Array("Go Back A Step - Manu", "Go to next step-Manu") -> (w92:bool[])
            n26 = Boolean Array To Number(Boolean array=w92) -> (number=w91:u32)
            n27 = case shown="1" w91 {
              tunnel: w90 -> [w99 w106 w116]
              tunnel: [w99 w105 w115] -> w89
              frame 0, Default {
              }
              frame 1 {
                n28 = Decrement(x=w106) -> (x-1=w104:T7)
                n29 = In Range and Coerce(upper limit=7, x=w104, lower limit=0) -> (coerced(x)=w102:u32, In Range?=w103:bool)
                n30 = case shown="False" w103 {
                  tunnel: w104 -> [_ w112]
                  tunnel: [w107 w112] -> w105
                  tunnel: w102 -> [w109 _]
                  frame False {
                    n31 = Less Than 0?(x=w109) -> (x < 0?=w108:bool)
                    n32 = case shown="False" w108 {
                      tunnel: [T7."Enter Part Number" ("lower limit") T7."Label Instructions" ("lower limit")] -> w107
                      frame False {
                      }
                      frame True {
                      }
                    }
                  }
                  frame True {
                  }
                }
              }
              frame 2 {
                n33 = Increment(x=w116) -> (x+1=w119:T7)
                n34 = In Range and Coerce(upper limit=7, x=w119, lower limit=0) -> (coerced(x)=w117:u32, In Range?=w118:bool)
                n35 = case shown="True" w118 {
                  tunnel: w119 -> [_ w125]
                  tunnel: [w120 w125] -> w115
                  tunnel: w117 -> [w122 _]
                  frame False {
                    n36 = Less Than 0?(x=w122) -> (x < 0?=w121:bool)
                    n37 = case shown="False" w121 {
                      tunnel: [T7."Enter Part Number" ("lower limit") T7."Label Instructions" ("lower limit")] -> w120
                      frame False {
                      }
                      frame True {
                      }
                    }
                  }
                  frame True {
                  }
                }
              }
            }
            n38 = property on="Manufacturing Tab Instructions" class="TabCtl (strict)"(error in=w95, "Value"=w89) -> (error out=w97:errorcluster)  [unwired: 1 in, 1 out]
          }
          event "Go Back A Step - Insp", "Go to next step-Insp": Value Change {
            n39 = event-data() -> ()  [unwired: 1 in, 6 out]
            n40 = property on="Inspection Tab Instructions" class="TabCtl (strict)"(error in=w134) -> (error out=w133:errorcluster, "Value"=w131:T20)  [unwired: 1 in, 1 out]
            n41 = Build Array("Go Back A Step - Insp", "Go to next step-Insp") -> (w130:bool[])
            n42 = Boolean Array To Number(Boolean array=w130) -> (number=w128:u32)
            n43 = case shown="2" w128 {
              tunnel: w131 -> [w136 w143 w153]
              tunnel: [w136 w142 w152] -> w126
              frame 0, Default {
              }
              frame 1 {
                n44 = Decrement(x=w143) -> (x-1=w141:T20)
                n45 = In Range and Coerce(upper limit=7, x=w141, lower limit=0) -> (coerced(x)=w139:u32, In Range?=w140:bool)
                n46 = case shown="False" w140 {
                  tunnel: w141 -> [_ w149]
                  tunnel: [w144 w149] -> w142
                  tunnel: w139 -> [w146 _]
                  frame False {
                    n47 = Less Than 0?(x=w146) -> (x < 0?=w145:bool)
                    n48 = case shown="False" w145 {
                      tunnel: [T20."Enter Part Number" ("Inspection Tab Instructions") T20."Inspect Labels" ("Inspection Tab Instructions")] -> w144
                      frame False {
                      }
                      frame True {
                      }
                    }
                  }
                  frame True {
                  }
                }
              }
              frame 2 {
                n49 = Increment(x=w153) -> (x+1=w156:T20)
                n50 = In Range and Coerce(upper limit=7, x=w156, lower limit=0) -> (coerced(x)=w154:u32, In Range?=w155:bool)
                n51 = case shown="False" w155 {
                  tunnel: w156 -> [_ w162]
                  tunnel: [w157 w162] -> w152
                  tunnel: w154 -> [w159 _]
                  frame False {
                    n52 = Less Than 0?(x=w159) -> (x < 0?=w158:bool)
                    n53 = case shown="False" w158 {
                      tunnel: [T20."Inspect Labels" ("Inspection Tab Instructions") T20."Enter Part Number" ("Inspection Tab Instructions")] -> w157
                      frame False {
                      }
                      frame True {
                      }
                    }
                  }
                  frame True {
                  }
                }
              }
            }
            n54 = property on="Inspection Tab Instructions" class="TabCtl (strict)"(error in=w133, "Value"=w126) -> (error out=w132:errorcluster)  [unwired: 1 in, 1 out]
          }
          event Value Change {
            n55 = event-data() -> ()  [unwired: 1 in, 6 out]
            n56 = property on="Manufacturing Tab Instructions" class="TabCtl (strict)"(error in=w166) -> (error out=w165:errorcluster, "Value"=w164:T7)  [unwired: 1 in, 1 out]
            n57 = case shown="\"Visual Inspection Instruction\"" w164 {
              tunnel: w165 -> [w169 w171 w173 w175 w177 w179 w181]
              tunnel: [w168 w170 w172 w174 w176 w178 w180] -> w163
              frame "Enter Part Number", Default {
                n58 = invoke on="Manufacturing-Part Number" class="Str" method="Reinit To Default"(error in=w169) -> (error out=w168:errorcluster)  [unwired: 2 in, 2 out]
              }
              frame "Get Material Instructions" {
                n59 = invoke on="Manufacturing-Mat" class="Clust (strict)" method="Reinit To Default"(error in=w171) -> (error out=w170:errorcluster)  [unwired: 2 in, 2 out]
              }
              frame "Visual Inspection Instruction" {
                n60 = invoke on="Manufacturing-VisualInsp" class="Clust (strict)" method="Reinit To Default"(error in=w173) -> (error out=w172:errorcluster)  [unwired: 2 in, 2 out]
              }
              frame "Assemble Material as Required" {
                n61 = invoke on="Manufacturing-Assemble" class="Clust (strict)" method="Reinit To Default"(error in=w175) -> (error out=w174:errorcluster)  [unwired: 2 in, 2 out]
              }
              frame "Laser Cutting Instructions" {
                n62 = invoke on="Manufacturing-Laser" class="Clust (strict)" method="Reinit To Default"(error in=w177) -> (error out=w176:errorcluster)  [unwired: 2 in, 2 out]
              }
              frame "Cleaning Instructions" {
                n63 = invoke on="Manufacturing-Cleaning" class="Clust (strict)" method="Reinit To Default"(error in=w179) -> (error out=w178:errorcluster)  [unwired: 2 in, 2 out]
              }
              frame "Label Instructions" {
                n64 = invoke on="Manufacturing-Label" class="Clust (strict)" method="Reinit To Default"(error in=w181) -> (error out=w180:errorcluster)  [unwired: 2 in, 2 out]
              }
            }
          }
          event Value Change {
            n65 = event-data() -> ()  [unwired: 1 in, 6 out]
            n66 = property on="Inspection Tab Instructions" class="TabCtl (strict)"(error in=w185) -> (error out=w183:errorcluster, "Value"=w184:T20)  [unwired: 1 in, 1 out]
            n67 = case shown="\"Inspect Labels\"" w184 {
              tunnel: w183 -> [w188 w190 w192 w194 w196 w198 w200]
              tunnel: [w187 w189 w191 w193 w195 w197 w199] -> w182
              frame "Enter Part Number", Default {
                n68 = invoke on="Inspection Part Number" class="Str" method="Reinit To Default"(error in=w188) -> (error out=w187:errorcluster)  [unwired: 2 in, 2 out]
              }
              frame "Visually Inspect" {
                n69 = invoke on="Inspect-Visually Inspect" class="Clust (strict)" method="Reinit To Default"(error in=w190) -> (error out=w189:errorcluster)  [unwired: 2 in, 2 out]
              }
              frame "Certified Material" {
                n70 = invoke on="Inspect-Certified Material" class="Clust (strict)" method="Reinit To Default"(error in=w192) -> (error out=w191:errorcluster)  [unwired: 2 in, 2 out]
              }
              frame "XY Dimensions" {
                n71 = invoke on="Inspect-XY Dimensions" class="Clust (strict)" method="Reinit To Default"(error in=w194) -> (error out=w193:errorcluster)  [unwired: 2 in, 2 out]
              }
              frame "Measure Create Cert" {
                n72 = invoke on="Inspect-Measure Create Cert" class="Clust (strict)" method="Reinit To Default"(error in=w196) -> (error out=w195:errorcluster)  [unwired: 2 in, 2 out]
              }
              frame "Quantity Passed or Failed" {
                n73 = invoke on="Inspect-Qty P/F" class="Clust (strict)" method="Reinit To Default"(error in=w198) -> (error out=w197:errorcluster)  [unwired: 2 in, 2 out]
              }
              frame "Inspect Labels" {
                n74 = invoke on="Inspect-Inspect Labels" class="Clust (strict)" method="Reinit To Default"(error in=w200) -> (error out=w199:errorcluster)  [unwired: 2 in, 2 out]
              }
            }
          }
          event Value Change {
            n75 = event-data() -> ()  [unwired: 1 in, 6 out]
            n76 = invoke on="General Step Instruction" class="Clust (strict)" method="Reinit To Default"(error in=w202) -> (error out=w204:errorcluster)  [unwired: 2 in, 2 out]
            n77 = invoke on="General Process Name*" class="Str" method="Reinit To Default"(error in=w204) -> (error out=w203:errorcluster)  [unwired: 2 in, 2 out]
            n78 = invoke on="Step Number*" class="DigNum (strict)" method="Reinit To Default"(error in=w203) -> (error out=w201:errorcluster)  [unwired: 2 in, 2 out]
          }
          event Value Change {
            n79 = event-data() -> ()  [unwired: 1 in, 6 out]
            n80 = Build Array("Create Manufacturing Instruction", "Update Manufacturing Instruction", "Load Manufacturing Instruction", "Delete Manufacturing Instruction") -> (w220:T19[])
            n81 = Boolean Array To Number(Boolean array=w220) -> (number=w221:u32)
            n82 = case shown="8" w221 {
              tunnel: w226 -> [w228 w232 w237 w242 w249]
              tunnel: w225 -> [w229 w234 w239 w244 w247]
              tunnel: [w229 w233 w238 w243 w250] -> w211
              tunnel: [w228 w232 w237 w242 w249] -> w219
              tunnel: [w227 w230 w235 w240 w245] -> w207
              tunnel: "Manufacturing-Part Number" -> [w227 w230 w235 w240 _]
              frame 0, Default {
              }
              frame 1 {
                n83 = call "FTW-Actor-AddJob-Next.vi"("Add Next in Job Queue"="ActorDB: Create a Manufacturing Instruction", "FTW Actor Instance"=w234) -> ("FTW Actor Instance out"=w233:refnum<class "ERP-CreateInstructions.lvclass">)  [unwired: 2 in]
              }
              frame 2 {
                n84 = call "FTW-Actor-AddJob-Next.vi"("Add Next in Job Queue"="ActorDB: Update a Manufacturing Instruction", "FTW Actor Instance"=w239) -> ("FTW Actor Instance out"=w238:refnum<class "ERP-CreateInstructions.lvclass">)  [unwired: 2 in]
              }
              frame 4 {
                n85 = call "FTW-Actor-AddJob-Next.vi"("Add Next in Job Queue"="ActorDB: Load a Manufacturing Instruction", "FTW Actor Instance"=w244) -> ("FTW Actor Instance out"=w243:refnum<class "ERP-CreateInstructions.lvclass">)  [unwired: 2 in]
              }
              frame 8 {
                n86 = Unbundle By Name(w247) -> ("Manufacturing Tree - Instruction Sets"=w246:refnum<vi>)
                n87 = call "FTW-Actor-AddJob-Next.vi"("Add Next in Job Queue"="ActorDB: Delete a Manufacturing Instruction", "FTW Actor Instance"=w247) -> ("FTW Actor Instance out"=w250:refnum<class "ERP-CreateInstructions.lvclass">)  [unwired: 2 in]
                n88 = property class="Tree (strict)"(reference=w246) -> ("Value"=w245:string)  [unwired: 1 in, 2 out]
              }
            }
            n89 = Build Array("Manufacturing-Mat", "Manufacturing-VisualInsp", "Manufacturing-Assemble", "Manufacturing-Laser", "Manufacturing-Cleaning", "Manufacturing-Label") -> (w212:T34)
            n90 = Bundle("Value"=w207, w212) -> (w209:T35)  [unwired: 1 in]
            n91 = Bundle By Name(cluster=w211, "Manufacturing Cluster"=w209) -> (w210:refnum<class "ERP-CreateInstructions.lvclass">)
          }
          event Value Change {
            n92 = event-data() -> ()  [unwired: 1 in, 6 out]
            n93 = call "FTW-Actor-AddJob-Next.vi"("Add Next in Job Queue"="GI: Choose Manufacturing General Instruction", "FTW Actor Instance"=w252) -> ("FTW Actor Instance out"=w251:refnum<class "ERP-CreateInstructions.lvclass">)  [unwired: 2 in]
          }
          event Value Change {
            n94 = event-data() -> ()  [unwired: 1 in, 6 out]
            n95 = call "FTW-Actor-AddJob-Next.vi"("Add Next in Job Queue"="GI: Choose Inspection General Instruction", "FTW Actor Instance"=w256) -> ("FTW Actor Instance out"=w255:refnum<class "ERP-CreateInstructions.lvclass">)  [unwired: 2 in]
          }
          event Value Change {
            n96 = event-data() -> ()  [unwired: 1 in, 6 out]
            n97 = Build Array("Create Inspection Instruction", "Update Inspection Instruction", "Load Inspection Instruction", "Delete Inspection Instruction") -> (w279:T19[])
            n98 = Boolean Array To Number(Boolean array=w279) -> (number=w272:u32)
            n99 = case shown="8" w272 {
              tunnel: w274 -> [w281 w285 w290 w295 w302]
              tunnel: w275 -> [w282 w287 w292 w297 w300]
              tunnel: [w282 w286 w291 w296 w303] -> w261
              tunnel: [w281 w285 w290 w295 w302] -> w273
              tunnel: "Inspection Part Number" -> [w280 w283 w288 w293 _]
              tunnel: [w280 w283 w288 w293 w298] -> w259
              frame 0, Default {
              }
              frame 1 {
                n100 = call "FTW-Actor-AddJob-Next.vi"("Add Next in Job Queue"="ActorDB: Create a Inspection Instruction", "FTW Actor Instance"=w287) -> ("FTW Actor Instance out"=w286:refnum<class "ERP-CreateInstructions.lvclass">)  [unwired: 2 in]
              }
              frame 2 {
                n101 = call "FTW-Actor-AddJob-Next.vi"("Add Next in Job Queue"="ActorDB: Update a Inspection Instruction", "FTW Actor Instance"=w292) -> ("FTW Actor Instance out"=w291:refnum<class "ERP-CreateInstructions.lvclass">)  [unwired: 2 in]
              }
              frame 4 {
                n102 = call "FTW-Actor-AddJob-Next.vi"("Add Next in Job Queue"="ActorDB: Load a Inspection Instruction", "FTW Actor Instance"=w297) -> ("FTW Actor Instance out"=w296:refnum<class "ERP-CreateInstructions.lvclass">)  [unwired: 2 in]
              }
              frame 8 {
                n103 = Unbundle By Name(w300) -> ("Inspection Tree - Instruction Sets"=w299:refnum<vi>)
                n104 = property class="Tree (strict)"(reference=w299) -> ("Value"=w298:string)  [unwired: 1 in, 2 out]
                n105 = call "FTW-Actor-AddJob-Next.vi"("Add Next in Job Queue"="ActorDB: Delete a Inspection Instruction", "FTW Actor Instance"=w300) -> ("FTW Actor Instance out"=w303:refnum<class "ERP-CreateInstructions.lvclass">)  [unwired: 2 in]
              }
            }
            n106 = Build Array("Inspect-Visually Inspect", "Inspect-Certified Material", "Inspect-XY Dimensions", "Inspect-Measure Create Cert", "Inspect-Qty P/F", "Inspect-Inspect Labels") -> (w269:T36)
            n107 = Bundle("Value"=w259, w269) -> (w263:T37)  [unwired: 1 in]
            n108 = Bundle By Name(cluster=w261, "Inspection cluster"=w263) -> (w271:refnum<class "ERP-CreateInstructions.lvclass">)
          }
          event "Manufacturing Tree - Instruction Sets": Double Click {
            n109 = event-data() -> ()  [unwired: 1 in, 10 out]
            n110 = call "FTW-Actor-AddJob-Next.vi"("Add Next in Job Queue"="Data: Load Double Click Manu Instruction", "FTW Actor Instance"=w306) -> ("FTW Actor Instance out"=w305:refnum<class "ERP-CreateInstructions.lvclass">)  [unwired: 2 in]
          }
          event "Inspection Tree - Instruction Sets": Double Click {
            n111 = event-data() -> ()  [unwired: 1 in, 10 out]
            n112 = call "FTW-Actor-AddJob-Next.vi"("Add Next in Job Queue"="Data: Load Double Click Inspection Instruction", "FTW Actor Instance"=w309) -> ("FTW Actor Instance out"=w308:refnum<class "ERP-CreateInstructions.lvclass">)  [unwired: 2 in]
          }
          event Value Change {
            n113 = event-data() -> ()  [unwired: 1 in, 6 out]
            n114 = Build Array("Refresh Manufacturing Tree", "Refresh Inspection Tree", "Refresh General Tree") -> (w317:T5[])
            n115 = Boolean Array To Number(Boolean array=w317) -> (number=w316:u32)
            n116 = case shown="1" w316 {
              tunnel: w313 -> [w321 w324 w328 w332]
              tunnel: w315 -> [w322 w326 w330 w334]
              tunnel: [w322 w325 w329 w333] -> w314
              tunnel: [w321 w324 w328 w332] -> w312
              frame 0, Default {
              }
              frame 1 {
                n117 = call "FTW-Actor-AddJob-Next.vi"("Add Next in Job Queue"="Tree: Populate Manufacturing", "FTW Actor Instance"=w326) -> ("FTW Actor Instance out"=w325:refnum<class "ERP-CreateInstructions.lvclass">)  [unwired: 2 in]
              }
              frame 2 {
                n118 = call "FTW-Actor-AddJob-Next.vi"("Add Next in Job Queue"="Tree: Populate Inspection", "FTW Actor Instance"=w330) -> ("FTW Actor Instance out"=w329:refnum<class "ERP-CreateInstructions.lvclass">)  [unwired: 2 in]
              }
              frame 4 {
                n119 = call "FTW-Actor-AddJob-Next.vi"("Add Next in Job Queue"="Tree: Populate General", "FTW Actor Instance"=w334) -> ("FTW Actor Instance out"=w333:refnum<class "ERP-CreateInstructions.lvclass">)  [unwired: 2 in]
              }
            }
          }
          event Value Change {
            n120 = event-data() -> ()  [unwired: 1 in, 6 out]
            n121 = Build Array("Clear All Manu\nSteps", "Clear All Inspection\nSteps") -> (w340:T18[])
            n122 = Boolean Array To Number(Boolean array=w340) -> (number=w339:u32)
            n123 = case shown="2" w339 {
              tunnel: w337 -> [w343 w352 w361]
              tunnel: [w343 w344 w353] -> w338
              frame 0, Default {
              }
              frame 1 {
                n124 = invoke on="Manufacturing-Part Number" class="Str" method="Reinit To Default"(error in=w352) -> (error out=w351:errorcluster)  [unwired: 2 in, 2 out]
                n125 = invoke on="Manufacturing-Mat" class="Clust (strict)" method="Reinit To Default"(error in=w352) -> (error out=w350:errorcluster)  [unwired: 2 in, 2 out]
                n126 = invoke on="Manufacturing-VisualInsp" class="Clust (strict)" method="Reinit To Default"(error in=w352) -> (error out=w349:errorcluster)  [unwired: 2 in, 2 out]
                n127 = invoke on="Manufacturing-Assemble" class="Clust (strict)" method="Reinit To Default"(error in=w352) -> (error out=w347:errorcluster)  [unwired: 2 in, 2 out]
                n128 = invoke on="Manufacturing-Laser" class="Clust (strict)" method="Reinit To Default"(error in=w352) -> (error out=w348:errorcluster)  [unwired: 2 in, 2 out]
                n129 = invoke on="Manufacturing-Cleaning" class="Clust (strict)" method="Reinit To Default"(error in=w352) -> (error out=w346:errorcluster)  [unwired: 2 in, 2 out]
                n130 = invoke on="Manufacturing-Label" class="Clust (strict)" method="Reinit To Default"(error in=w352) -> (error out=w345:errorcluster)  [unwired: 2 in, 2 out]
                n131 = Merge Errors(w351, w350, w349, w347, w348, w346, w345) -> (w344:errorcluster)
              }
              frame 2 {
                n132 = invoke on="Inspection Part Number" class="Str" method="Reinit To Default"(error in=w361) -> (error out=w360:errorcluster)  [unwired: 2 in, 2 out]
                n133 = invoke on="Inspect-Visually Inspect" class="Clust (strict)" method="Reinit To Default"(error in=w361) -> (error out=w359:errorcluster)  [unwired: 2 in, 2 out]
                n134 = invoke on="Inspect-Certified Material" class="Clust (strict)" method="Reinit To Default"(error in=w361) -> (error out=w358:errorcluster)  [unwired: 2 in, 2 out]
                n135 = invoke on="Inspect-XY Dimensions" class="Clust (strict)" method="Reinit To Default"(error in=w361) -> (error out=w357:errorcluster)  [unwired: 2 in, 2 out]
                n136 = invoke on="Inspect-Measure Create Cert" class="Clust (strict)" method="Reinit To Default"(error in=w361) -> (error out=w356:errorcluster)  [unwired: 2 in, 2 out]
                n137 = invoke on="Inspect-Qty P/F" class="Clust (strict)" method="Reinit To Default"(error in=w361) -> (error out=w355:errorcluster)  [unwired: 2 in, 2 out]
                n138 = invoke on="Inspect-Inspect Labels" class="Clust (strict)" method="Reinit To Default"(error in=w361) -> (error out=w354:errorcluster)  [unwired: 2 in, 2 out]
                n139 = Merge Errors(w360, w359, w358, w357, w356, w355, w354) -> (w353:errorcluster)
              }
            }
            n140 = Merge Errors(w338, w337) -> (w336:errorcluster)
          }
          event Value Change {
            n141 = event-data() -> ()  [unwired: 1 in, 1 out]
            n142 = Build Array("Create General Instruction", "Update General Instruction", "Delete General Instruction") -> (w370:T19[])
            n143 = Boolean Array To Number(Boolean array=w370) -> (number=w365:u32)
            n144 = case shown="4" w365 {
              tunnel: w371 -> [w379 w383 w388 w395]
              tunnel: w372 -> [w380 w385 w390 w393]
              tunnel: [w380 w384 w389 w396] -> w367
              tunnel: [w379 w383 w388 w395] -> w366
              tunnel: [w378 w381 w386 w391] -> w363
              tunnel: "General Process Name*" -> [w378 w381 w386 _]
              frame 0, Default {
              }
              frame 1 {
                n145 = call "FTW-Actor-AddJob-Next.vi"("Add Next in Job Queue"="ActorDB: Create a General Instruction", "FTW Actor Instance"=w385) -> ("FTW Actor Instance out"=w384:refnum<class "ERP-CreateInstructions.lvclass">)  [unwired: 2 in]
              }
              frame 2 {
                n146 = call "FTW-Actor-AddJob-Next.vi"("Add Next in Job Queue"="ActorDB: Update a General Instruction", "FTW Actor Instance"=w390) -> ("FTW Actor Instance out"=w389:refnum<class "ERP-CreateInstructions.lvclass">)  [unwired: 2 in]
              }
              frame 4 {
                n147 = Unbundle By Name(w393) -> ("General Tree - Instruction Sets"=w392:refnum<vi>)
                n148 = call "FTW-Actor-AddJob-Next.vi"("Add Next in Job Queue"="ActorDB: Delete a General Instruction", "FTW Actor Instance"=w393) -> ("FTW Actor Instance out"=w396:refnum<class "ERP-CreateInstructions.lvclass">)  [unwired: 2 in]
                n149 = property class="Tree (strict)"(reference=w392) -> ("Value"=w391:string)  [unwired: 1 in, 2 out]
              }
            }
            n150 = Bundle(cluster=T30 {"Manufacturing-Part Number"="", 0.0, "Manufacturing-Label"={"Label Instructions"="", "Path for Picture Label"=path "", "Path for Picture Label 2"=path "", "Path for Picture Label 3"=path "", "Path for Picture Label 4"=path "", "Path for Picture Label 5"=path "", "Path for Picture Label 6"=path "", "Path for Picture Label 7"=path ""}}, "Manufacturing-Part Number"=w363, "Step Number*", "Manufacturing-Label"="General Step Instruction") -> (w374:T30)
            n151 = Bundle By Name(cluster=w367, "General Instruction"=w374) -> (w373:refnum<class "ERP-CreateInstructions.lvclass">)
          }
          event "General Tree - Instruction Sets": Double Click {
            n152 = event-data() -> ()  [unwired: 1 in, 10 out]
            n153 = call "FTW-Actor-AddJob-Next.vi"("Add Next in Job Queue"="Data: Load Double Click General Instruction", "FTW Actor Instance"=w398) -> ("FTW Actor Instance out"=w397:refnum<class "ERP-CreateInstructions.lvclass">)  [unwired: 2 in]
          }
          event "Stop Button": Value Change {
            n154 = event-data() -> ()  [unwired: 1 in, 6 out]
            n155 = call "FTW-Actor-BeginShutdownSequence.vi"("FTW Actor Instance"=w402) -> ("FTW Actor Instance out"=w401:refnum<class "ERP-CreateInstructions.lvclass">)  [unwired: 3 in]
          }
          event Panel Close? {
            n156 = event-data() -> ()  [unwired: 1 in, 1 out]
            n157 = call "FTW-Actor-BeginShutdownSequence.vi"("FTW Actor Instance"=w405) -> ("FTW Actor Instance out"=w404:refnum<class "ERP-CreateInstructions.lvclass">)  [unwired: 3 in]
            n158 = event-data("Discard?"=TRUE) -> ()  [unwired: 1 in, 1 out]
          }
        }
      }
      frame "FTW: Initialize" {
        w414 = refnum<event-registration> refnum  # Additional Registration Types
        n159 = property on="Tab Control -Main" class="TabCtl (strict)"(error in=w410, "Value"=T31."Welcome Page" ("Tab Control -TI Plates")) -> (error out=w409:errorcluster)  [unwired: 1 in, 1 out]
        n160 = disable-structure shown="Disabled" {
          disable-tunnel: w409 -> [w421 w422]
          disable-tunnel: [w420 w422] -> w408
          frame Disabled {
            n161 = invoke class="VI" method="Default Vals.Reinit All"(error in=w421) -> (error out=w420:errorcluster)  [unwired: 2 in, 2 out]
          }
          frame Enabled {
          }
        }
        n162 = call "PCert-ConfigPageNF-InRequests.vi"("error in (no error)"=w408, "ERP-ConfigPageNF in"=w417) -> ("error out"=w415:errorcluster, "Incoming Requests"=w413:refnum<event-registration>, "ERP-ConfigPageNF out"=w416:refnum<class "ERP-CreateInstructions.lvclass">)  [unwired: 7 in]
        n163 = Bundle("Incoming Requests"=w413, "Additional Registration Types"=w414) -> (w412:T38)  [unwired: 1 in]
        n164 = call-dynamic "FTW-Actor-Initialized.vi"("FTW Actor Instance"=w416, "error in"=w415) -> ("FTW Actor Instance out"=w419:refnum<class "ERP-CreateInstructions.lvclass">, "error out"=w418:errorcluster)  [unwired: 12 in]
      }
      frame "FTW:Initialize State Data" {
        n165 = control-ref of="Manufacturing Tree - Instruction Sets"() -> (w426:refnum<vi>)
        n166 = control-ref of="General Tree - Instruction Sets"() -> (w423:refnum<vi>)
        n167 = control-ref of="Inspection Tree - Instruction Sets"() -> (w424:refnum<vi>)
        n168 = call "Instruction-SupportStateData.vi"("ERP-CreateInstructions in"=w427, "Manufacturing Tree - Instruction Sets"=w426, "Inspection Tree - Instruction Sets"=w424, "General Tree - Instruction Sets"=w423) -> ("ERP-CreateInstructions out"=w425:refnum<class "ERP-CreateInstructions.lvclass">)  [unwired: 15 in]
      }
      frame "FTW: Error Handler" {
        n169 = call-dynamic "FTW-Actor-HandleError.vi"("FTW Actor Instance"=w433, "error in"=w432) -> ("FTW Actor Instance out"=w431:refnum<class "ERP-CreateInstructions.lvclass">, "error out"=w430:errorcluster)  [unwired: 11 in, 1 out]
      }
      frame "FTW: Unknown Job", Default {
        n170 = call-dynamic "FTW-Actor-UnknownJob.vi"("FTW Actor Instance"=w437, "Unknown Job"=w435, "error in"=w439) -> ("FTW Actor Instance out"=w436:refnum<class "ERP-CreateInstructions.lvclass">, "error out"=w438:errorcluster)  [unwired: 11 in]
      }
      frame "FTW: Shutdown" {
        n171 = call "PCert-ConfigPageNF-CloseActorConn.vi"("error in (no error)"=w443, "ERP-ConfigPageNF in"=w444) -> ("error out"=w442:errorcluster, "ERP-ConfigPageNF out"=w441:refnum<class "ERP-CreateInstructions.lvclass">)  [unwired: 8 in]
        n172 = Unbundle(w448) -> ("Incoming Requests"=w447:refnum<event-registration>)  [unwired: 1 out]
        n173 = Unregister For Events(event registration refnum=w447) -> (error out=w445:errorcluster)  [unwired: 1 in]
        n174 = Merge Errors(w442, w445) -> (w446:errorcluster)
      }
      frame "FTW Sequence: Shutdown" {
        w449 = "FTW: Shutdown"  # Shutdown Sequence
        n175 = call "FTW-Actor-AddJob-Next.vi"("Add Next in Job Queue"=w449, "FTW Actor Instance"=w451) -> ("FTW Actor Instance out"=w450:refnum<class "ERP-CreateInstructions.lvclass">)  [unwired: 2 in]
      }
      frame "==== Actor-Specific Job Sequences ====" {
        w454 = ""  # Job Sequence
        n176 = call "FTW-Actor-AddJob-Next.vi"("Add Next in Job Queue"=w454, "FTW Actor Instance"=w456) -> ("FTW Actor Instance out"=w455:refnum<class "ERP-CreateInstructions.lvclass">)  [unwired: 2 in]
      }
      frame "==== Actor-Specific Jobs ====" {
      }
      frame "ActorDB: Create a Manufacturing Instruction" {
        n177 = Unbundle By Name(w463) -> ("Manufacturing-Part Number"=w476:string, "Arrary of Steps"=w475:T39)
        n178 = Bundle(cluster=T32 {"Manufacturing-Part Number"="", "Array of Cluster Data"=[], "Type of Insert"=0}, "Manufacturing-Part Number"=w476, "Array of Cluster Data"=w475, "Type of Insert"=0) -> (w481:T32)
        n179 = Flatten To String(anything=w481, error in (no error)=w462) -> (data string=w479:string, error out=w480:errorcluster)  [unwired: 2 in, 1 out]
        n180 = call "FTW-STR-Encode-Base64.vi"("Input"=w479, "Direction"=enum16{"Encode", "Decode"}."Encode") -> ("Output"=w478:string)
        n181 = call "LVtoJSON-DBInsert.vi"("Payload"=w478, "Update All"=TRUE, "error in"=w480, "Table"="ManuInstructions") -> ("error out"=w471:errorcluster, "Output JSON Object"=w470:string)  [unwired: 6 in]
        n182 = call "PCert-ConfigPageNF-AskDB.vi"("Timeout"=500, "error in (no error)"=w471, "Request Body"=w470, "Request Header"="InsertInstructions" ("Message Header"), "ERP-ConfigPageNF in"=w463) -> ("error out"=w467:errorcluster, "ERP-ConfigPageNF out"=w468:refnum<class "ERP-CreateInstructions.lvclass">, "Raw Data From DB"=w469:string[][])  [unwired: 2 in, 2 out]
        n183 = call "Tree-RefreshManufacturingTree.vi"("Raw Data From DB Actor"=w469, "error in (no error)"=w467, "ERP-CreateInstructions in"=w468) -> ("error out"=w465:errorcluster, "ERP-CreateInstructions out"=w466:refnum<class "ERP-CreateInstructions.lvclass">)  [unwired: 7 in]
      }
      frame "ActorDB: Create a Inspection Instruction" {
        n184 = Unbundle By Name(w486) -> ("Inspection-Part Number"=w498:string, "Arrary of Steps"=w497:T34)
        n185 = Bundle(cluster=T32 {"Manufacturing-Part Number"="", "Array of Cluster Data"=[], "Type of Insert"=0}, "Manufacturing-Part Number"=w498, "Array of Cluster Data"=w497, "Type of Insert"=0) -> (w503:T32)
        n186 = Flatten To String(anything=w503, error in (no error)=w485) -> (data string=w501:string, error out=w502:errorcluster)  [unwired: 2 in, 1 out]
        n187 = call "FTW-STR-Encode-Base64.vi"("Input"=w501, "Direction"=enum16{"Encode", "Decode"}."Encode") -> ("Output"=w500:string)
        n188 = call "LVtoJSON-DBInsert.vi"("Payload"=w500, "Update All"=TRUE, "error in"=w502, "Table"="InspectInstructions") -> ("error out"=w489:errorcluster, "Output JSON Object"=w488:string)  [unwired: 6 in]
        n189 = call "PCert-ConfigPageNF-AskDB.vi"("Timeout"=500, "error in (no error)"=w489, "Request Body"=w488, "Request Header"="InsertInstructions" ("Message Header"), "ERP-ConfigPageNF in"=w486) -> ("error out"=w496:errorcluster, "ERP-ConfigPageNF out"=w490:refnum<class "ERP-CreateInstructions.lvclass">, "Raw Data From DB"=w495:string[][])  [unwired: 2 in, 2 out]
        n190 = call "Tree-RefreshInspectionTree.vi"("Raw Data From DB Actor"=w495, "error in (no error)"=w496, "ERP-CreateInstructions in"=w490) -> ("error out"=w491:errorcluster, "ERP-CreateInstructions out"=w492:refnum<class "ERP-CreateInstructions.lvclass">)  [unwired: 7 in]
      }
      frame "ActorDB: Create a General Instruction" {
        n191 = Unbundle By Name(w515) -> ("General-Part Number"=w523:string, "Step Number"=w521:dbl, "Manufacturing-Label"=w520:T40)
        n192 = Bundle(cluster=T33 {"Manufacturing-Part Number"="", "Step Number"=0.0, "Gernal Cluster Data"={"Label Instructions"="", "Path for Picture Label"=path "", "Path for Picture Label 2"=path "", "Path for Picture Label 3"=path "", "Path for Picture Label 4"=path "", "Path for Picture Label 5"=path "", "Path for Picture Label 6"=path "", "Path for Picture Label 7"=path ""}, "Type of Insert"=0}, "Manufacturing-Part Number"=w523, "Step Number"=w521, "Gernal Cluster Data"=w520, "Type of Insert"=1) -> (w528:T33)
        n193 = Flatten To String(anything=w528, error in (no error)=w519) -> (data string=w526:string, error out=w527:errorcluster)  [unwired: 2 in, 1 out]
        n194 = call "FTW-STR-Encode-Base64.vi"("Input"=w526, "Direction"=enum16{"Encode", "Decode"}."Encode") -> ("Output"=w525:string)
        n195 = call "LVtoJSON-DBInsert.vi"("Payload"=w525, "Update All"=TRUE, "error in"=w527, "Table"="GeneralInstructions") -> ("error out"=w514:errorcluster, "Output JSON Object"=w513:string)  [unwired: 6 in]
        n196 = call "PCert-ConfigPageNF-AskDB.vi"("Timeout"=500, "error in (no error)"=w514, "Request Body"=w513, "Request Header"="InsertInstructions" ("Message Header"), "ERP-ConfigPageNF in"=w515) -> ("error out"=w512:errorcluster, "ERP-ConfigPageNF out"=w508:refnum<class "ERP-CreateInstructions.lvclass">, "Raw Data From DB"=w509:string[][])  [unwired: 2 in, 2 out]
        n197 = call "Tree-RefreshGeneralTree.vi"("Raw Data From DB Actor"=w509, "error in (no error)"=w512, "ERP-CreateInstructions in"=w508) -> ("error out"=w510:errorcluster, "ERP-CreateInstructions out"=w511:refnum<class "ERP-CreateInstructions.lvclass">)  [unwired: 7 in]
      }
      frame "ActorDB: Update a Manufacturing Instruction" {
        n198 = Unbundle By Name(w533) -> ("Manufacturing-Part Number"=w551:string, "Arrary of Steps"=w550:T39)
        n199 = Bundle(cluster=T32 {"Manufacturing-Part Number"="", "Array of Cluster Data"=[], "Type of Insert"=0}, "Manufacturing-Part Number"=w551, "Array of Cluster Data"=w550) -> (w553:T32)  [unwired: 1 in]
        n200 = Flatten To String(anything=w553, error in (no error)=w532) -> (data string=w552:string, error out=w546:errorcluster)  [unwired: 2 in, 1 out]
        n201 = call "FTW-STR-Encode-Base64.vi"("Input"=w552, "Direction"=enum16{"Encode", "Decode"}."Encode") -> ("Output"=w547:string)
        n202 = call "LVtoJSON-DBUpdateAll.vi"("Datatype"=3, "Payload"=w547, "Update All"=TRUE, "error in"=w546, "SQL Statement"="Where PartNumber ='%1$s' and Step ='%2$s'", "Table"="ManuInstructions") -> ("error out"=w540:errorcluster, "Output JSON Object"=w541:string)  [unwired: 4 in]
        n203 = call "PCert-ConfigPageNF-AskDB.vi"("Timeout"=500, "error in (no error)"=w540, "Request Body"=w541, "Request Header"="UpdateInstructions" ("Message Header"), "ERP-ConfigPageNF in"=w533) -> ("error out"=w538:errorcluster, "ERP-ConfigPageNF out"=w537:refnum<class "ERP-CreateInstructions.lvclass">, "Raw Data From DB"=w536:string[][])  [unwired: 2 in, 2 out]
        n204 = call "Tree-RefreshManufacturingTree.vi"("Raw Data From DB Actor"=w536, "error in (no error)"=w538, "ERP-CreateInstructions in"=w537) -> ("error out"=w534:errorcluster, "ERP-CreateInstructions out"=w535:refnum<class "ERP-CreateInstructions.lvclass">)  [unwired: 7 in]
      }
      frame "ActorDB: Update a Inspection Instruction" {
        n205 = Unbundle By Name(w557) -> ("Inspection-Part Number"=w575:string, "Arrary of Steps"=w574:T34)
        n206 = Bundle(cluster=T32 {"Manufacturing-Part Number"="", "Array of Cluster Data"=[], "Type of Insert"=0}, "Manufacturing-Part Number"=w575, "Array of Cluster Data"=w574) -> (w577:T32)  [unwired: 1 in]
        n207 = Flatten To String(anything=w577, error in (no error)=w556) -> (data string=w576:string, error out=w570:errorcluster)  [unwired: 2 in, 1 out]
        n208 = call "FTW-STR-Encode-Base64.vi"("Input"=w576, "Direction"=enum16{"Encode", "Decode"}."Encode") -> ("Output"=w571:string)
        n209 = call "LVtoJSON-DBUpdateAll.vi"("Datatype"=3, "Payload"=w571, "Update All"=TRUE, "error in"=w570, "SQL Statement"="Where PartNumber ='%1$s' and Step ='%2$s'", "Table"="InspectInstructions") -> ("error out"=w564:errorcluster, "Output JSON Object"=w563:string)  [unwired: 4 in]
        n210 = call "PCert-ConfigPageNF-AskDB.vi"("Timeout"=500, "error in (no error)"=w564, "Request Body"=w563, "Request Header"="UpdateInstructions" ("Message Header"), "ERP-ConfigPageNF in"=w557) -> ("error out"=w560:errorcluster, "ERP-ConfigPageNF out"=w562:refnum<class "ERP-CreateInstructions.lvclass">, "Raw Data From DB"=w561:string[][])  [unwired: 2 in, 2 out]
        n211 = call "Tree-RefreshInspectionTree.vi"("Raw Data From DB Actor"=w561, "error in (no error)"=w560, "ERP-CreateInstructions in"=w562) -> ("error out"=w558:errorcluster, "ERP-CreateInstructions out"=w559:refnum<class "ERP-CreateInstructions.lvclass">)  [unwired: 7 in]
      }
      frame "ActorDB: Update a General Instruction" {
        n212 = Unbundle By Name(w587) -> ("General-Part Number"=w593:string, "Step Number"=w592:dbl, "Manufacturing-Label"=w591:T40)
        n213 = Bundle(cluster=T30 {"Manufacturing-Part Number"="", 0.0, "Manufacturing-Label"={"Label Instructions"="", "Path for Picture Label"=path "", "Path for Picture Label 2"=path "", "Path for Picture Label 3"=path "", "Path for Picture Label 4"=path "", "Path for Picture Label 5"=path "", "Path for Picture Label 6"=path "", "Path for Picture Label 7"=path ""}}, "Manufacturing-Part Number"=w593, w592, "Manufacturing-Label"=w591) -> (w602:T30)
        n214 = Flatten To String(anything=w602, error in (no error)=w590) -> (data string=w601:string, error out=w597:errorcluster)  [unwired: 2 in, 1 out]
        n215 = call "FTW-STR-Encode-Base64.vi"("Input"=w601, "Direction"=enum16{"Encode", "Decode"}."Encode") -> ("Output"=w598:string)
        n216 = call "LVtoJSON-DBUpdateAll.vi"("Datatype"=3, "Payload"=w598, "Update All"=TRUE, "error in"=w597, "SQL Statement"="Where GeneralProcessName ='%1$s' and StepNumber ='%2$s'", "Table"="GeneralInstructions") -> ("error out"=w585:errorcluster, "Output JSON Object"=w586:string)  [unwired: 4 in]
        n217 = call "PCert-ConfigPageNF-AskDB.vi"("Timeout"=500, "error in (no error)"=w585, "Request Body"=w586, "Request Header"="UpdateInstructions" ("Message Header"), "ERP-ConfigPageNF in"=w587) -> ("error out"=w582:errorcluster, "ERP-ConfigPageNF out"=w584:refnum<class "ERP-CreateInstructions.lvclass">, "Raw Data From DB"=w583:string[][])  [unwired: 2 in, 2 out]
        n218 = call "Tree-RefreshGeneralTree.vi"("Raw Data From DB Actor"=w583, "error in (no error)"=w582, "ERP-CreateInstructions in"=w584) -> ("error out"=w580:errorcluster, "ERP-CreateInstructions out"=w581:refnum<class "ERP-CreateInstructions.lvclass">)  [unwired: 7 in]
      }
      frame "ActorDB: Load a Manufacturing Instruction" {
        # "Load all steps with the current part number"
        n219 = call "Manufacturing-LoadAllSteps.vi"("error in (no error)"=w615, "ERP-CreateInstructions in"=w614) -> ("error out"=w611:errorcluster, "All Part# Info"=w612:T41, "ERP-CreateInstructions out"=w613:refnum<class "ERP-CreateInstructions.lvclass">, "Part Number"=w610:string)  [unwired: 6 in]
        n220 = property on="Manufacturing-Part Number" class="Str"(error in=w611, "Value"=w610) -> (error out=w608:errorcluster)  [unwired: 1 in, 1 out]
        n221 = for {
          tunnel: w612 -> [w619] mode=indexing
          tunnel: w608 -> [w618]
          tunnel: [w617] -> w609 mode=indexing
          i -> [w620]
          n222 = case shown="5" w620 {
            tunnel: w619 -> [w623 w626 w629 w632 w635 w638]
            tunnel: w618 -> [w622 w625 w628 w631 w634 w637]
            tunnel: [w621 w624 w627 w630 w633 w636] -> w617
            frame 0, Default {
              n223 = property on="Manufacturing-Mat" class="Clust (strict)"(error in=w622, "Value"=w623) -> (error out=w621:errorcluster)  [unwired: 1 in, 1 out]
            }
            frame 1 {
              n224 = property on="Manufacturing-VisualInsp" class="Clust (strict)"(error in=w625, "Value"=w626) -> (error out=w624:errorcluster)  [unwired: 1 in, 1 out]
            }
            frame 2 {
              n225 = property on="Manufacturing-Assemble" class="Clust (strict)"(error in=w628, "Value"=w629) -> (error out=w627:errorcluster)  [unwired: 1 in, 1 out]
            }
            frame 3 {
              n226 = property on="Manufacturing-Laser" class="Clust (strict)"(error in=w631, "Value"=w632) -> (error out=w630:errorcluster)  [unwired: 1 in, 1 out]
            }
            frame 4 {
              n227 = property on="Manufacturing-Cleaning" class="Clust (strict)"(error in=w634, "Value"=w635) -> (error out=w633:errorcluster)  [unwired: 1 in, 1 out]
            }
            frame 5 {
              n228 = property on="Manufacturing-Label" class="Clust (strict)"(error in=w637, "Value"=w638) -> (error out=w636:errorcluster)  [unwired: 1 in, 1 out]
            }
          }
        }
        n229 = Merge Errors(w608, w609) -> (w607:errorcluster)
        n230 = property on="Manufacturing Tab Instructions" class="TabCtl (strict)"(error in=w607, "Value"=T7."Enter Part Number" ("Manufacturing Tab Instructions")) -> (error out=w606:errorcluster)  [unwired: 1 in, 1 out]
      }
      frame "ActorDB: Load a Inspection Instruction" {
        # "Load all steps with the current part number"
        n231 = call "Inspection-LoadAllSteps.vi"("error in (no error)"=w648, "ERP-CreateInstructions in"=w647) -> ("error out"=w643:errorcluster, "All Part# Info"=w645:T41, "ERP-CreateInstructions out"=w646:refnum<class "ERP-CreateInstructions.lvclass">, "Part Number"=w644:string)  [unwired: 6 in]
        n232 = property on="Inspection Part Number" class="Str"(error in=w643, "Value"=w644) -> (error out=w642:errorcluster)  [unwired: 1 in, 1 out]
        n233 = for {
          tunnel: w645 -> [w653] mode=indexing
          tunnel: w642 -> [w652]
          tunnel: [w651] -> w649 mode=indexing
          i -> [w654]
          n234 = case shown="4" w654 {
            tunnel: w653 -> [w657 w660 w663 w666 w669 w672]
            tunnel: w652 -> [w656 w659 w662 w665 w668 w671]
            tunnel: [w655 w658 w661 w664 w667 w670] -> w651
            frame 0, Default {
              n235 = property on="Inspect-Visually Inspect" class="Clust (strict)"(error in=w656, "Value"=w657) -> (error out=w655:errorcluster)  [unwired: 1 in, 1 out]
            }
            frame 1 {
              n236 = property on="Inspect-Certified Material" class="Clust (strict)"(error in=w659, "Value"=w660) -> (error out=w658:errorcluster)  [unwired: 1 in, 1 out]
            }
            frame 2 {
              n237 = property on="Inspect-XY Dimensions" class="Clust (strict)"(error in=w662, "Value"=w663) -> (error out=w661:errorcluster)  [unwired: 1 in, 1 out]
            }
            frame 3 {
              n238 = property on="Inspect-Measure Create Cert" class="Clust (strict)"(error in=w665, "Value"=w666) -> (error out=w664:errorcluster)  [unwired: 1 in, 1 out]
            }
            frame 4 {
              n239 = property on="Inspect-Qty P/F" class="Clust (strict)"(error in=w668, "Value"=w669) -> (error out=w667:errorcluster)  [unwired: 1 in, 1 out]
            }
            frame 5 {
              n240 = property on="Inspect-Inspect Labels" class="Clust (strict)"(error in=w671, "Value"=w672) -> (error out=w670:errorcluster)  [unwired: 1 in, 1 out]
            }
          }
        }
        n241 = Merge Errors(w642, w649) -> (w640:errorcluster)
        n242 = property on="Inspection Tab Instructions" class="TabCtl (strict)"(error in=w640, "Value"=T20."Enter Part Number" ("Inspection Tab Instructions")) -> (error out=w639:errorcluster)  [unwired: 1 in, 1 out]
      }
      frame "ActorDB: Delete a Inspection Instruction" {
        n243 = Unbundle By Name(w681) -> ("Inspection-Part Number"=w692:string, "Arrary of Steps"=w691:T34)
        n244 = Bundle(cluster=T32 {"Manufacturing-Part Number"="", "Array of Cluster Data"=[], "Type of Insert"=0}, "Manufacturing-Part Number"=w692, "Array of Cluster Data"=w691, "Type of Insert"=0) -> (w694:T32)
        n245 = Flatten To String(anything=w694, error in (no error)=w684) -> (data string=w693:string, error out=w676:errorcluster)  [unwired: 2 in, 1 out]
        n246 = call "FTW-STR-Encode-Base64.vi"("Input"=w693, "Direction"=enum16{"Encode", "Decode"}."Encode") -> ("Output"=w673:string)
        n247 = call "LVtoJSON-DBUpdateAll.vi"("Datatype"=3, "Payload"=w673, "Update All"=TRUE, "error in"=w676, "SQL Statement"="Where PartNumber ='%1$s'", "Table"="InspectInstructions") -> ("error out"=w675:errorcluster, "Output JSON Object"=w674:string)  [unwired: 4 in]
        n248 = call "PCert-ConfigPageNF-AskDB.vi"("Timeout"=500, "error in (no error)"=w675, "Request Body"=w674, "Request Header"="DeleteInstruction" ("Message Header"), "ERP-ConfigPageNF in"=w681) -> ("error out"=w690:errorcluster, "ERP-ConfigPageNF out"=w686:refnum<class "ERP-CreateInstructions.lvclass">, "Raw Data From DB"=w689:string[][])  [unwired: 2 in, 2 out]
        n249 = call "Tree-RefreshInspectionTree.vi"("Raw Data From DB Actor"=w689, "error in (no error)"=w690, "ERP-CreateInstructions in"=w686) -> ("error out"=w682:errorcluster, "ERP-CreateInstructions out"=w683:refnum<class "ERP-CreateInstructions.lvclass">)  [unwired: 7 in]
      }
      frame "ActorDB: Delete a Manufacturing Instruction" {
        n250 = Unbundle By Name(w711) -> ("Manufacturing-Part Number"=w717:string, "Arrary of Steps"=w716:T39)
        n251 = Bundle(cluster=T32 {"Manufacturing-Part Number"="", "Array of Cluster Data"=[], "Type of Insert"=0}, "Manufacturing-Part Number"=w717, "Array of Cluster Data"=w716, "Type of Insert"=0) -> (w719:T32)
        n252 = Flatten To String(anything=w719, error in (no error)=w712) -> (data string=w718:string, error out=w706:errorcluster)  [unwired: 2 in, 1 out]
        n253 = call "FTW-STR-Encode-Base64.vi"("Input"=w718, "Direction"=enum16{"Encode", "Decode"}."Encode") -> ("Output"=w703:string)
        n254 = call "LVtoJSON-DBUpdateAll.vi"("Datatype"=3, "Payload"=w703, "Update All"=TRUE, "error in"=w706, "SQL Statement"="Where PartNumber ='%1$s'", "Table"="ManuInstructions") -> ("error out"=w705:errorcluster, "Output JSON Object"=w704:string)  [unwired: 4 in]
        n255 = call "PCert-ConfigPageNF-AskDB.vi"("Timeout"=500, "error in (no error)"=w705, "Request Body"=w704, "Request Header"="DeleteInstruction" ("Message Header"), "ERP-ConfigPageNF in"=w711) -> ("error out"=w701:errorcluster, "ERP-ConfigPageNF out"=w702:refnum<class "ERP-CreateInstructions.lvclass">, "Raw Data From DB"=w700:string[][])  [unwired: 2 in, 2 out]
        n256 = call "Tree-RefreshManufacturingTree.vi"("Raw Data From DB Actor"=w700, "error in (no error)"=w701, "ERP-CreateInstructions in"=w702) -> ("error out"=w698:errorcluster, "ERP-CreateInstructions out"=w699:refnum<class "ERP-CreateInstructions.lvclass">)  [unwired: 7 in]
      }
      frame "ActorDB: Delete a General Instruction" {
        w730 = ":" ("regular expression")
        n257 = Unbundle By Name(w746) -> ("General Tree - Instruction Sets"=w734:refnum<vi>)
        n258 = property class="Tree (strict)"(reference=w734, error in=w733) -> (error out=w732:errorcluster, "Value"=w729:string)  [unwired: 1 out]
        n259 = Match Pattern(string=w729, regular expression=w730) -> (match substring=w731:string)  [unwired: 1 in, 3 out]
        n260 = Equal?(x=w731, y=w730) -> (x = y?=w728:bool)
        n261 = case shown="True" w728 {
          tunnel: ["Where GeneralProcessName ='%1$s'" ("SQL Statement") "Where GeneralProcessName ='%1$s' and StepNumber ='%2$s'" ("SQL Statement")] -> w742
          frame False {
          }
          frame True {
          }
        }
        n262 = Bundle(cluster=T32 {"Manufacturing-Part Number"="", "Array of Cluster Data"=[], "Type of Insert"=0}, "Manufacturing-Part Number"=w729, "Type of Insert"=0) -> (w735:T32)  [unwired: 1 in]
        n263 = Flatten To String(anything=w735, error in (no error)=w732) -> (data string=w749:string, error out=w741:errorcluster)  [unwired: 2 in, 1 out]
        n264 = call "FTW-STR-Encode-Base64.vi"("Input"=w749, "Direction"=enum16{"Encode", "Decode"}."Encode") -> ("Output"=w738:string)
        n265 = call "LVtoJSON-DBUpdateAll.vi"("Datatype"=3, "Payload"=w738, "Update All"=TRUE, "error in"=w741, "SQL Statement"=w742, "Table"="GeneralInstructions") -> ("error out"=w740:errorcluster, "Output JSON Object"=w739:string)  [unwired: 4 in]
        n266 = call "PCert-ConfigPageNF-AskDB.vi"("Timeout"=500, "error in (no error)"=w740, "Request Body"=w739, "Request Header"="DeleteInstruction" ("Message Header"), "ERP-ConfigPageNF in"=w746) -> ("error out"=w724:errorcluster, "ERP-ConfigPageNF out"=w726:refnum<class "ERP-CreateInstructions.lvclass">, "Raw Data From DB"=w725:string[][])  [unwired: 2 in, 2 out]
        n267 = call "Tree-RefreshGeneralTree.vi"("Raw Data From DB Actor"=w725, "error in (no error)"=w724, "ERP-CreateInstructions in"=w726) -> ("error out"=w723:errorcluster, "ERP-CreateInstructions out"=w727:refnum<class "ERP-CreateInstructions.lvclass">)  [unwired: 7 in]
      }
      frame "========Tree Jobs============" {
      }
      frame "Tree: Populate Manufacturing" {
        w772 = ""
        n268 = call "JSON-ActorCommand.vi"("Payload"=w772, "error in"=w769, "Reply Command"="Refresh Tree - Manufacturing" ("Value"), "SQL Statement"=w772, "Table"="ManuInstructions") -> ("error out"=w765:errorcluster, "Output JSON Object"=w764:string)  [unwired: 5 in]
        n269 = call "PCert-ConfigPageNF-AskDB.vi"("Timeout"=2000, "error in (no error)"=w765, "Request Body"=w764, "Request Header"="Query" ("Message Header"), "ERP-ConfigPageNF in"=w766) -> ("error out"=w761:errorcluster, "ERP-ConfigPageNF out"=w762:refnum<class "ERP-CreateInstructions.lvclass">, "Raw Data From DB"=w763:string[][])  [unwired: 2 in, 2 out]
        n270 = call "Tree-RefreshManufacturingTree.vi"("Raw Data From DB Actor"=w763, "error in (no error)"=w761, "ERP-CreateInstructions in"=w762) -> ("error out"=w759:errorcluster, "ERP-CreateInstructions out"=w760:refnum<class "ERP-CreateInstructions.lvclass">)  [unwired: 7 in]
        n271 = call <vilib>:"Wait n mSec.vi"("error in (no error)"=w759, "Milliseconds to Wait (500)"=u32 125) -> ("error out"=w757:errorcluster)  [unwired: 13 in]
      }
      frame "Tree: Populate Inspection" {
        w789 = ""
        n272 = call "JSON-ActorCommand.vi"("Payload"=w789, "error in"=w786, "Reply Command"="Refresh Tree - Inspection" ("Value"), "SQL Statement"=w789, "Table"="InspectInstructions") -> ("error out"=w781:errorcluster, "Output JSON Object"=w782:string)  [unwired: 5 in]
        n273 = call "PCert-ConfigPageNF-AskDB.vi"("Timeout"=2000, "error in (no error)"=w781, "Request Body"=w782, "Request Header"="Query" ("Message Header"), "ERP-ConfigPageNF in"=w783) -> ("error out"=w779:errorcluster, "ERP-ConfigPageNF out"=w778:refnum<class "ERP-CreateInstructions.lvclass">, "Raw Data From DB"=w780:string[][])  [unwired: 2 in, 2 out]
        n274 = call "Tree-RefreshInspectionTree.vi"("Raw Data From DB Actor"=w780, "error in (no error)"=w779, "ERP-CreateInstructions in"=w778) -> ("error out"=w775:errorcluster, "ERP-CreateInstructions out"=w777:refnum<class "ERP-CreateInstructions.lvclass">)  [unwired: 7 in]
        n275 = call <vilib>:"Wait n mSec.vi"("error in (no error)"=w775, "Milliseconds to Wait (500)"=u32 125) -> ("error out"=w774:errorcluster)  [unwired: 13 in]
      }
      frame "Tree: Populate General" {
        w806 = ""
        n276 = call "JSON-ActorCommand.vi"("Payload"=w806, "error in"=w803, "Reply Command"="Refresh Tree - General" ("Value"), "SQL Statement"=w806, "Table"="GeneralInstructions") -> ("error out"=w799:errorcluster, "Output JSON Object"=w798:string)  [unwired: 5 in]
        n277 = call "PCert-ConfigPageNF-AskDB.vi"("Timeout"=2000, "error in (no error)"=w799, "Request Body"=w798, "Request Header"="Query" ("Message Header"), "ERP-ConfigPageNF in"=w800) -> ("error out"=w797:errorcluster, "ERP-ConfigPageNF out"=w796:refnum<class "ERP-CreateInstructions.lvclass">, "Raw Data From DB"=w795:string[][])  [unwired: 2 in, 2 out]
        n278 = call "Tree-RefreshGeneralTree.vi"("Raw Data From DB Actor"=w795, "error in (no error)"=w797, "ERP-CreateInstructions in"=w796) -> ("error out"=w792:errorcluster, "ERP-CreateInstructions out"=w794:refnum<class "ERP-CreateInstructions.lvclass">)  [unwired: 7 in]
        n279 = call <vilib>:"Wait n mSec.vi"("error in (no error)"=w792, "Milliseconds to Wait (500)"=u32 125) -> ("error out"=w791:errorcluster)  [unwired: 13 in]
      }
      frame "=========Data============" {
      }
      frame "Data: Get General Instructions" {
      }
      frame "Data: Load Double Click Manu Instruction" {
        n280 = call "Manufacturing-LoadSingleStep.vi"("error in (no error)"=w821, "ERP-CreateInstructions in"=w820) -> ("error out"=w815:errorcluster, "Step#"=w819:i32, "ERP-CreateInstructions out"=w818:refnum<class "ERP-CreateInstructions.lvclass">, "Cluster for Step"=w817:T42, "Part Number"=w816:string)  [unwired: 5 in]
        n281 = case shown="6" w819 {
          selector: w819 -> [_ w826 w833 w840 w847 w854 w861]
          tunnel: w817 -> [_ w830 w837 w844 w851 w858 w865]
          tunnel: w816 -> [_ w828 w835 w842 w849 w856 w864]
          tunnel: w815 -> [w823 w825 w832 w839 w846 w853 w862]
          tunnel: [w823 w827 w834 w841 w848 w855 w863] -> w814
          frame 0, Default {
          }
          frame 1 {
            n282 = property on="Manufacturing \nTab Instructions" class="TabCtl (strict)"(error in=w825, "Value"=w826) -> (error out=w824:errorcluster)  [unwired: 1 in, 1 out]
            n283 = property on="Manufacturing-Mat" class="Clust (strict)"(error in=w824, "Value"=w830) -> (error out=w829:errorcluster)  [unwired: 1 in, 1 out]
            n284 = property on="Manufacturing-Part Number" class="Str"(error in=w829, "Value"=w828) -> (error out=w827:errorcluster)  [unwired: 1 in, 1 out]
          }
          frame 2 {
            n285 = property on="Manufacturing \nTab Instructions" class="TabCtl (strict)"(error in=w832, "Value"=w833) -> (error out=w831:errorcluster)  [unwired: 1 in, 1 out]
            n286 = property on="Manufacturing-VisualInsp" class="Clust (strict)"(error in=w831, "Value"=w837) -> (error out=w836:errorcluster)  [unwired: 1 in, 1 out]
            n287 = property on="Manufacturing-Part Number" class="Str"(error in=w836, "Value"=w835) -> (error out=w834:errorcluster)  [unwired: 1 in, 1 out]
          }
          frame 3 {
            n288 = property on="Manufacturing \nTab Instructions" class="TabCtl (strict)"(error in=w839, "Value"=w840) -> (error out=w838:errorcluster)  [unwired: 1 in, 1 out]
            n289 = property on="Manufacturing-Assemble" class="Clust (strict)"(error in=w838, "Value"=w844) -> (error out=w843:errorcluster)  [unwired: 1 in, 1 out]
            n290 = property on="Manufacturing-Part Number" class="Str"(error in=w843, "Value"=w842) -> (error out=w841:errorcluster)  [unwired: 1 in, 1 out]
          }
          frame 4 {
            n291 = property on="Manufacturing \nTab Instructions" class="TabCtl (strict)"(error in=w846, "Value"=w847) -> (error out=w845:errorcluster)  [unwired: 1 in, 1 out]
            n292 = property on="Manufacturing-Laser" class="Clust (strict)"(error in=w845, "Value"=w851) -> (error out=w850:errorcluster)  [unwired: 1 in, 1 out]
            n293 = property on="Manufacturing-Part Number" class="Str"(error in=w850, "Value"=w849) -> (error out=w848:errorcluster)  [unwired: 1 in, 1 out]
          }
          frame 5 {
            n294 = property on="Manufacturing \nTab Instructions" class="TabCtl (strict)"(error in=w853, "Value"=w854) -> (error out=w852:errorcluster)  [unwired: 1 in, 1 out]
            n295 = property on="Manufacturing-Cleaning" class="Clust (strict)"(error in=w852, "Value"=w858) -> (error out=w857:errorcluster)  [unwired: 1 in, 1 out]
            n296 = property on="Manufacturing-Part Number" class="Str"(error in=w857, "Value"=w856) -> (error out=w855:errorcluster)  [unwired: 1 in, 1 out]
          }
          frame 6 {
            n297 = property on="Manufacturing \nTab Instructions" class="TabCtl (strict)"(error in=w862, "Value"=w861) -> (error out=w860:errorcluster)  [unwired: 1 in, 1 out]
            n298 = property on="Manufacturing-Label" class="Clust (strict)"(error in=w860, "Value"=w865) -> (error out=w859:errorcluster)  [unwired: 1 in, 1 out]
            n299 = property on="Manufacturing-Part Number" class="Str"(error in=w859, "Value"=w864) -> (error out=w863:errorcluster)  [unwired: 1 in, 1 out]
          }
        }
      }
      frame "Data: Load Double Click Inspection Instruction" {
        n300 = call "Inspection-LoadSingleStep.vi"("error in (no error)"=w871, "ERP-CreateInstructions in"=w872) -> ("error out"=w866:errorcluster, "Step#"=w867:i32, "ERP-CreateInstructions out"=w868:refnum<class "ERP-CreateInstructions.lvclass">, "Cluster for Step"=w869:T43, "Part Number"=w870:string)  [unwired: 5 in]
        n301 = case shown="6" w867 {
          selector: w867 -> [_ w882 w888 w896 w903 w910 w917]
          tunnel: w869 -> [_ w880 w885 w892 w899 w906 w913]
          tunnel: w870 -> [_ w878 w887 w893 w900 w907 w915]
          tunnel: w866 -> [w875 w881 w889 w895 w902 w909 w916]
          tunnel: [w875 w876 w886 w894 w901 w908 w914] -> w873
          frame 0, Default {
          }
          frame 1 {
            n302 = property on="Inspection Tab Instructions" class="TabCtl (strict)"(error in=w881, "Value"=w882) -> (error out=w879:errorcluster)  [unwired: 1 in, 1 out]
            n303 = property on="Inspect-Visually Inspect" class="Clust (strict)"(error in=w879, "Value"=w880) -> (error out=w877:errorcluster)  [unwired: 1 in, 1 out]
            n304 = property on="Inspection Part Number" class="Str"(error in=w877, "Value"=w878) -> (error out=w876:errorcluster)  [unwired: 1 in, 1 out]
          }
          frame 2 {
            n305 = property on="Inspection Tab Instructions" class="TabCtl (strict)"(error in=w889, "Value"=w888) -> (error out=w884:errorcluster)  [unwired: 1 in, 1 out]
            n306 = property on="Inspect-Certified Material" class="Clust (strict)"(error in=w884, "Value"=w885) -> (error out=w883:errorcluster)  [unwired: 1 in, 1 out]
            n307 = property on="Inspection Part Number" class="Str"(error in=w883, "Value"=w887) -> (error out=w886:errorcluster)  [unwired: 1 in, 1 out]
          }
          frame 3 {
            n308 = property on="Inspection Tab Instructions" class="TabCtl (strict)"(error in=w895, "Value"=w896) -> (error out=w891:errorcluster)  [unwired: 1 in, 1 out]
            n309 = property on="Inspect-XY Dimensions" class="Clust (strict)"(error in=w891, "Value"=w892) -> (error out=w890:errorcluster)  [unwired: 1 in, 1 out]
            n310 = property on="Inspection Part Number" class="Str"(error in=w890, "Value"=w893) -> (error out=w894:errorcluster)  [unwired: 1 in, 1 out]
          }
          frame 4 {
            n311 = property on="Inspection Tab Instructions" class="TabCtl (strict)"(error in=w902, "Value"=w903) -> (error out=w898:errorcluster)  [unwired: 1 in, 1 out]
            n312 = property on="Inspect-Measure Create Cert" class="Clust (strict)"(error in=w898, "Value"=w899) -> (error out=w897:errorcluster)  [unwired: 1 in, 1 out]
            n313 = property on="Inspection Part Number" class="Str"(error in=w897, "Value"=w900) -> (error out=w901:errorcluster)  [unwired: 1 in, 1 out]
          }
          frame 5 {
            n314 = property on="Inspection Tab Instructions" class="TabCtl (strict)"(error in=w909, "Value"=w910) -> (error out=w905:errorcluster)  [unwired: 1 in, 1 out]
            n315 = property on="Inspect-Qty P/F" class="Clust (strict)"(error in=w905, "Value"=w906) -> (error out=w904:errorcluster)  [unwired: 1 in, 1 out]
            n316 = property on="Inspection Part Number" class="Str"(error in=w904, "Value"=w907) -> (error out=w908:errorcluster)  [unwired: 1 in, 1 out]
          }
          frame 6 {
            n317 = property on="Inspection Tab Instructions" class="TabCtl (strict)"(error in=w916, "Value"=w917) -> (error out=w912:errorcluster)  [unwired: 1 in, 1 out]
            n318 = property on="Inspect-Inspect Labels" class="Clust (strict)"(error in=w912, "Value"=w913) -> (error out=w911:errorcluster)  [unwired: 1 in, 1 out]
            n319 = property on="Inspection Part Number" class="Str"(error in=w911, "Value"=w915) -> (error out=w914:errorcluster)  [unwired: 1 in, 1 out]
          }
        }
      }
      frame "Data: Load Double Click General Instruction" {
        n320 = call "General-LoadSingleStep.vi"("error in (no error)"=w926, "ERP-CreateInstructions in"=w927) -> ("error out"=w924:errorcluster, "Step Number"=w923:string, "ERP-CreateInstructions out"=w928:refnum<class "ERP-CreateInstructions.lvclass">, "Cluster for Step"=w925:T44, "General Process Name"=w918:string)  [unwired: 5 in]
        n321 = property on="General Step Instruction" class="Clust (strict)"(error in=w924, "Value"=w925) -> (error out=w921:errorcluster)  [unwired: 1 in, 1 out]
        n322 = Fract/Exp String To Number(string=w923) -> (number=w922:dbl)  [unwired: 3 in, 1 out]
        n323 = property on="Step Number*" class="DigNum (strict)"(error in=w921, "Value"=w922) -> (error out=w920:errorcluster)  [unwired: 1 in, 1 out]
        n324 = property on="General Process Name*" class="Str"(error in=w920, "Value"=w918) -> (error out=w919:errorcluster)  [unwired: 1 in, 1 out]
      }
      frame "=========General Instructions=========" {
      }
      frame "GI: Choose Manufacturing General Instruction" {
        w938 = ""
        n325 = call "JSON-ActorCommand.vi"("Payload"=w938, "error in"=w936, "SQL Statement"=w938, "Table"="GeneralInstructions") -> ("error out"=w942:errorcluster, "Output JSON Object"=w943:string)  [unwired: 6 in]
        n326 = call "PCert-ConfigPageNF-AskDB.vi"("Timeout"=2000, "error in (no error)"=w942, "Request Body"=w943, "Request Header"="Query" ("Message Header"), "ERP-ConfigPageNF in"=w937) -> ("error out"=w935:errorcluster, "ERP-ConfigPageNF out"=w934:refnum<class "ERP-CreateInstructions.lvclass">, "Raw Data From DB"=w933:string[][])  [unwired: 2 in, 2 out]
        n327 = property on="Manufacturing Tab Instructions" class="TabCtl (strict)"(error in=w935) -> (error out=w946:errorcluster, "Value"=w947:T7)  [unwired: 1 in, 1 out]
        n328 = case shown="\"Visual Inspection Instruction\"" w947 {
          tunnel: w934 -> [w951 w957 w964 w972 w979 w986 w993]
          tunnel: w946 -> [w950 w958 w965 w971 w978 w985 w992]
          tunnel: [w951 w952 w959 w969 w976 w983 w990] -> w944
          tunnel: [w950 w954 w960 w966 w973 w980 w987] -> w945
          tunnel: w933 -> [_ w956 w963 w970 w977 w984 w991]
          frame "Enter Part Number", Default {
            n329 = One Button Dialog(message="You cannot choose a General Instruction for the part number. Each step for the part number has the option to choose a General Instruction") -> ()  [unwired: 1 in, 1 out]
          }
          frame "Get Material Instructions" {
            n330 = call "GenInstr-MainPopUp.vi"("Raw Data From DB Actor"=w956, "error in (no error)"=w958, "ERP-CreateInstructions in"=w957) -> ("error out"=w955:errorcluster, "ERP-CreateInstructions out"=w952:refnum<class "ERP-CreateInstructions.lvclass">, "Selected Instruction"=w953:string)  [unwired: 6 in]
            n331 = property on="General Instruction" class="Str"(error in=w955, "Value"=w953) -> (error out=w954:errorcluster)  [unwired: 1 in, 1 out]
          }
          frame "Visual Inspection Instruction" {
            n332 = call "GenInstr-MainPopUp.vi"("Raw Data From DB Actor"=w963, "error in (no error)"=w965, "ERP-CreateInstructions in"=w964) -> ("error out"=w961:errorcluster, "ERP-CreateInstructions out"=w959:refnum<class "ERP-CreateInstructions.lvclass">, "Selected Instruction"=w962:string)  [unwired: 6 in]
            n333 = property on="General Instruction" class="Str"(error in=w961, "Value"=w962) -> (error out=w960:errorcluster)  [unwired: 1 in, 1 out]
          }
          frame "Assemble Material as Required" {
            n334 = call "GenInstr-MainPopUp.vi"("Raw Data From DB Actor"=w970, "error in (no error)"=w971, "ERP-CreateInstructions in"=w972) -> ("error out"=w967:errorcluster, "ERP-CreateInstructions out"=w969:refnum<class "ERP-CreateInstructions.lvclass">, "Selected Instruction"=w968:string)  [unwired: 6 in]
            n335 = property on="General Instruction" class="Str"(error in=w967, "Value"=w968) -> (error out=w966:errorcluster)  [unwired: 1 in, 1 out]
          }
          frame "Laser Cutting Instructions" {
            n336 = call "GenInstr-MainPopUp.vi"("Raw Data From DB Actor"=w977, "error in (no error)"=w978, "ERP-CreateInstructions in"=w979) -> ("error out"=w974:errorcluster, "ERP-CreateInstructions out"=w976:refnum<class "ERP-CreateInstructions.lvclass">, "Selected Instruction"=w975:string)  [unwired: 6 in]
            n337 = property on="General Instruction" class="Str"(error in=w974, "Value"=w975) -> (error out=w973:errorcluster)  [unwired: 1 in, 1 out]
          }
          frame "Cleaning Instructions" {
            n338 = call "GenInstr-MainPopUp.vi"("Raw Data From DB Actor"=w984, "error in (no error)"=w985, "ERP-CreateInstructions in"=w986) -> ("error out"=w981:errorcluster, "ERP-CreateInstructions out"=w983:refnum<class "ERP-CreateInstructions.lvclass">, "Selected Instruction"=w982:string)  [unwired: 6 in]
            n339 = property on="General Instruction" class="Str"(error in=w981, "Value"=w982) -> (error out=w980:errorcluster)  [unwired: 1 in, 1 out]
          }
          frame "Label Instructions" {
            n340 = call "GenInstr-MainPopUp.vi"("Raw Data From DB Actor"=w991, "error in (no error)"=w992, "ERP-CreateInstructions in"=w993) -> ("error out"=w988:errorcluster, "ERP-CreateInstructions out"=w990:refnum<class "ERP-CreateInstructions.lvclass">, "Selected Instruction"=w989:string)  [unwired: 6 in]
            n341 = property on="General Instruction" class="Str"(error in=w988, "Value"=w989) -> (error out=w987:errorcluster)  [unwired: 1 in, 1 out]
          }
        }
      }
      frame "GI: Choose Inspection General Instruction" {
        w1003 = ""
        n342 = call "JSON-ActorCommand.vi"("Payload"=w1003, "error in"=w1001, "SQL Statement"=w1003, "Table"="GeneralInstructions") -> ("error out"=w1007:errorcluster, "Output JSON Object"=w1008:string)  [unwired: 6 in]
        n343 = call "PCert-ConfigPageNF-AskDB.vi"("Timeout"=2000, "error in (no error)"=w1007, "Request Body"=w1008, "Request Header"="Query" ("Message Header"), "ERP-ConfigPageNF in"=w1002) -> ("error out"=w995:errorcluster, "ERP-ConfigPageNF out"=w996:refnum<class "ERP-CreateInstructions.lvclass">, "Raw Data From DB"=w994:string[][])  [unwired: 2 in, 2 out]
        n344 = property on="Inspection Tab Instructions" class="TabCtl (strict)"(error in=w995) -> (error out=w999:errorcluster, "Value"=w1000:T20)  [unwired: 1 in, 1 out]
        n345 = case shown="\"Inspect Labels\"" w1000 {
          tunnel: w996 -> [w1012 w1018 w1025 w1033 w1040 w1047 w1054]
          tunnel: w999 -> [w1011 w1019 w1026 w1032 w1039 w1046 w1053]
          tunnel: [w1012 w1016 w1023 w1029 w1037 w1044 w1051] -> w998
          tunnel: [w1011 w1013 w1020 w1027 w1034 w1041 w1048] -> w997
          tunnel: w994 -> [_ w1017 w1024 w1031 w1038 w1045 w1052]
          frame "Enter Part Number", Default {
            n346 = One Button Dialog(message="You cannot choose a General Instruction for the part number. Each step for the part number has the option to choose a General Instruction") -> ()  [unwired: 1 in, 1 out]
          }
          frame "Visually Inspect" {
            n347 = call "GenInstr-MainPopUp.vi"("Raw Data From DB Actor"=w1017, "error in (no error)"=w1019, "ERP-CreateInstructions in"=w1018) -> ("error out"=w1014:errorcluster, "ERP-CreateInstructions out"=w1016:refnum<class "ERP-CreateInstructions.lvclass">, "Selected Instruction"=w1015:string)  [unwired: 6 in]
            n348 = property on="General Instruction" class="Str"(error in=w1014, "Value"=w1015) -> (error out=w1013:errorcluster)  [unwired: 1 in, 1 out]
          }
          frame "Certified Material" {
            n349 = call "GenInstr-MainPopUp.vi"("Raw Data From DB Actor"=w1024, "error in (no error)"=w1026, "ERP-CreateInstructions in"=w1025) -> ("error out"=w1021:errorcluster, "ERP-CreateInstructions out"=w1023:refnum<class "ERP-CreateInstructions.lvclass">, "Selected Instruction"=w1022:string)  [unwired: 6 in]
            n350 = property on="General Instruction" class="Str"(error in=w1021, "Value"=w1022) -> (error out=w1020:errorcluster)  [unwired: 1 in, 1 out]
          }
          frame "XY Dimensions" {
            n351 = call "GenInstr-MainPopUp.vi"("Raw Data From DB Actor"=w1031, "error in (no error)"=w1032, "ERP-CreateInstructions in"=w1033) -> ("error out"=w1028:errorcluster, "ERP-CreateInstructions out"=w1029:refnum<class "ERP-CreateInstructions.lvclass">, "Selected Instruction"=w1030:string)  [unwired: 6 in]
            n352 = property on="General Instruction" class="Str"(error in=w1028, "Value"=w1030) -> (error out=w1027:errorcluster)  [unwired: 1 in, 1 out]
          }
          frame "Measure Create Cert" {
            n353 = call "GenInstr-MainPopUp.vi"("Raw Data From DB Actor"=w1038, "error in (no error)"=w1039, "ERP-CreateInstructions in"=w1040) -> ("error out"=w1035:errorcluster, "ERP-CreateInstructions out"=w1037:refnum<class "ERP-CreateInstructions.lvclass">, "Selected Instruction"=w1036:string)  [unwired: 6 in]
            n354 = property on="General Instruction" class="Str"(error in=w1035, "Value"=w1036) -> (error out=w1034:errorcluster)  [unwired: 1 in, 1 out]
          }
          frame "Quantity Passed or Failed" {
            n355 = call "GenInstr-MainPopUp.vi"("Raw Data From DB Actor"=w1045, "error in (no error)"=w1046, "ERP-CreateInstructions in"=w1047) -> ("error out"=w1042:errorcluster, "ERP-CreateInstructions out"=w1044:refnum<class "ERP-CreateInstructions.lvclass">, "Selected Instruction"=w1043:string)  [unwired: 6 in]
            n356 = property on="General Instruction" class="Str"(error in=w1042, "Value"=w1043) -> (error out=w1041:errorcluster)  [unwired: 1 in, 1 out]
          }
          frame "Inspect Labels" {
            n357 = call "GenInstr-MainPopUp.vi"("Raw Data From DB Actor"=w1052, "error in (no error)"=w1053, "ERP-CreateInstructions in"=w1054) -> ("error out"=w1049:errorcluster, "ERP-CreateInstructions out"=w1051:refnum<class "ERP-CreateInstructions.lvclass">, "Selected Instruction"=w1050:string)  [unwired: 6 in]
            n358 = property on="General Instruction" class="Str"(error in=w1049, "Value"=w1050) -> (error out=w1048:errorcluster)  [unwired: 1 in, 1 out]
          }
        }
      }
    }
    n359 = call "FTW-Actor-CheckShutdown.vi"("FTW Actor Instance"=w16, "error in"=w14) -> ("FTW Actor Instance out"=w15:refnum<class "ERP-CreateInstructions.lvclass">, "Shutdown?"=w12:bool, "error out"=w13:errorcluster)  [unwired: 11 in]
  }
  n360 = call-dynamic "FTW-Actor-Destroy.vi"("FTW Actor Instance"=w9, "Force Destroy?"=TRUE, "error in"=w8) -> ("error out"=→"Error":errorcluster)  [unwired: 12 in]
